vi "Tclk FGV.vi"(8 "Action":T1(ring), 9 "Options":T5={"GetInfo"=TRUE, "Set Det A para"=TRUE, "Set WD"=FALSE, "Set Mag"=TRUE, "Set stig"=FALSE, "Set aln"=FALSE, "Display"=TRUE, "Save"=TRUE, "8-bit"=TRUE, "Detector A"=TRUE, "Detector B"=TRUE, "Detector C"=FALSE, "Detector D"=FALSE, "Inverse A"=FALSE, "Inverse B"=FALSE, "Inverse C"=FALSE, "Inverse D"=FALSE, "Inverse PNG"=FALSE, "Freeze"=TRUE, "PNG only"=FALSE, "Upload"=FALSE, "Delete after upload"=FALSE}, 10 "Scan Para":T3={"X resolution"=0, "Y resolution"=0, "X center (um)"=0.0, "Y center (um)"=0.0, "X size (V)"=0.0, "X size auto"=TRUE, "X stig"=0.0, "Y stig"=0.0, "X aln"=0.0, "Y aln"=0.0, "Scan rate (Hz)"=0, "Oversampling"=0, "Oversampling auto"=TRUE, "Frame line rampdown ratio"=0.0, "Pixel size (nm)"=0.0, "WD"=0.0} {"WD" format="%#_7g"; "Frame line rampdown ratio" min=-1 max=1 step=0.05 format="%.2g"; "Scan rate (Hz)" max=4000000 format="%.2e"}, 11 "HW Config":T4={"SEM X coil"="", "SEM Y coil"="", "Detectors"="", "Det min (V)"=-10.0, "Det max (V)"=10.0, "Eanable COM"=TRUE, "COM port"="", "Detector FIB-NI auto switch"="", "Machine Type"=0, "Machine ID"=""} {"Machine Type" items=["Feiss", "NVision"]}) -> (0 "Tclk handle valid":bool, 3 "Initialized handles":T2={"sessions out"=[], "SEM-X handle out"="", "SEM-Y handle out"="", "SEM-Y waveform handle out"=0, "Detectors handle out"="", "channels"="", "error out"={"status"=FALSE, "code"=0, "source"=""}, "Others"={"AO SampClk.MaxRate"=100000000.0, "AI SampClk.MaxRate"=100000000.0, "AO rate"=10000000.0, "Scan speed"=1, "Detector number"=2, "X min (V)"=-10.0, "X max (V)"=10.0, "X min index"=0, "X max index"=4095, "Y min (V)"=-10.0, "Y max (V)"=10.0, "AO multiline"=128, "Decimating factor"=8, "Total time"=0.9240575999999999, "Scan time (m)"=0.0, "Scan time (s)"=0.9240575999999999, "X resolution"=4096, "Y resolution"=2048, "X resolution with rampdown"=4512, "Oversampling"=10, "Y scan pts per line"=0, "Y scan pts per AO multiline"=0, "Small scan"=FALSE, "Y single line pattern"=[], "Detectors min record length"=0, "Waveform blocks"=16, "Repeat count"=1, "Waveform size"=1155072, "AI multiline"=256}} {"Others"."Scan time (s)" format="%.3f"; "Others"."Scan speed" scale=1.0..15.0; "Others"."AO rate" format="%#_3e"})   [LabVIEW 2018]
uses:
  <instrlib>/niFgen/niFgen.llb/niFgen Output Mode.ctl
  <instrlib>/niScope/Configure/Trigger/niScope Configure Trigger Software.vi
  <instrlib>/niFgen/niFgen.llb/niFgen Write Waveform.vi
  <instrlib>/niFgen/niFgen.llb/niFgen Create Waveform (DBL).vi
  <vilib>/regexp/Match Regular Expression.xnode
panel:
  out "Y min (V)":dbl=-10.0
  out "Y max (V)":dbl=10.0
  out "Detector number":u8=2
  out "X min index":i32
  out "X min (V)":dbl=-10.0
  out "X max index":i32=4095
  out "X max (V)":dbl=10.0
  out "Detector A":bool=TRUE
  out "Detector B":bool=TRUE
  out "Decimating factor":u16=8
  in  "Image fit to":u8(ring) items=["Width", "Height"]
  out "AO multiline":u32=128
  out "Total time":dbl=0.9240575999999999
  out "Y scan pattern":dbl[](array[numeric])
  out "Scan speed":u8(slide)=1 scale=1.0..15.0
  out "Scan time (s)":dbl=0.9240575999999999 format="%.3f"
  out "Scan time (m)":dbl
  out "AI multiline":u16=256
  out "Waveform size":u32=1155072
  out "Repeat count":u32=1
  out "Waveform blocks":u32=16
  out "Small scan":bool
  out "AI SampClk.MaxRate":dbl=100000000.0
  out "AO SampClk.MaxRate":dbl=100000000.0
  out "COM port":refnum<visa-resource-name>="COM1"
  out "X resolution":u32=4096
  out "Y resolution":u32=2048
  out "Scan rate (Hz)":u32=10000000
  out "Oversampling":u32=10
  out "Frame line rampdown ratio":sgl=0.1
  out "Pixel size (nm)":sgl=5.0
  out "WD":sgl=4.0
  out "Det min (V)":dbl=-10.0
  out "Det max (V)":dbl=10.0
  out "X stig":sgl
  out "Y stig":sgl
  out "Detector FIB-NI auto switch":tag="FIB/port0/line0"
  out "SEM X coil":refnum<k15>="SEM-X"
  out "SEM Y coil":refnum<k15>="SEM-Y"
  out "Detectors":refnum<k15>="Detectors"
  out "Y scan rate factor":u8=8
  out "Gain":dbl=10.0
  out "X resolution with rampdown":i32=4512
  out "X single line pattern":dbl[](graph)
  out "Y single line pattern":dbl[](graph)=[-0.5, -0.49951148021494873, -0.4990229604298974, -0.4985344406448461, -0.4980459208597948, -0.49755740107474355, -0.49706888128969223, -0.4965803615046409, -0.49609184171958964, -0.4956033219345384, -0.49511480214948705, -0.49462628236443573, -0.49413776257938447, -0.4936492427943332, -0.4931607230092819, -0.49267220322423055, -0.4921836834391793, -0.491695163654128, -0.4912066438690767, -0.4907181240840254, -0.4902296042989741, -0.48974108451392284, -0.4892525647288715, -0.4887640449438202, -0.48827552515876893, -0.48778700537371766, -0.48729848558866634, -0.486809965803615, -0.48632144601856375, -0.4858329262335125, -0.48534440644846116, -0.48485588666340984, -0.4843673668783586, -0.4838788470933073, -0.483390327308256, -0.48290180752320466, -0.4824132877381534, -0.48192476795310213, -0.4814362481680508, -0.4809477283829995, -0.4804592085979482, -0.47997068881289695, -0.47948216902784563, -0.4789936492427943, -0.47850512945774304, -0.4780166096726918, -0.47752808988764045, -0.4770395701025891, -0.47655105031753786, -0.4760625305324866, -0.47557401074743527, -0.47508549096238395, -0.4745969711773327, -0.4741084513922814, -0.4736199316072301, -0.47313141182217877, -0.4726428920371275, -0.47215437225207624, -0.4716658524670249, -0.4711773326819736, -0.4706888128969223, -0.47020029311187106, -0.46971177332681974, -0.4692232535417684, -0.46873473375671715, -0.4682462139716659, -0.46775769418661456, -0.46726917440156324, -0.46678065461651197, -0.4662921348314607, -0.4658036150464094, -0.46531509526135806, -0.4648265754763068, -0.4643380556912555, -0.4638495359062042, -0.4633610161211529, -0.4628724963361016, -0.46238397655105035, -0.461895456765999, -0.4614069369809477, -0.46091841719589643, -0.46042989741084517, -0.45994137762579385, -0.4594528578407425, -0.45896433805569126, -0.45847581827064, -0.45798729848558867, -0.45749877870053735, -0.4570102589154861, -0.4565217391304348, -0.4560332193453835, -0.45554469956033217, -0.4550561797752809, -0.45456765999022963, -0.4540791402051783, -0.453590620420127, -0.4531021006350757, -0.45261358085002446, -0.45212506106497313, -0.4516365412799218, -0.45114802149487054, -0.4506595017098193, -0.45017098192476795, -0.44968246213971663, -0.44919394235466537, -0.4487054225696141, -0.4482169027845628, -0.44772838299951145, -0.4472398632144602, -0.4467513434294089, -0.4462628236443576, -0.4457743038593063, -0.445285784074255, -0.44479726428920374, -0.4443087445041524, -0.4438202247191011, -0.44333170493404983, -0.44284318514899856, -0.44235466536394724, -0.4418661455788959, -0.44137762579384465, -0.4408891060087934, -0.44040058622374206, -0.43991206643869074, -0.4394235466536395, -0.4389350268685882, -0.4384465070835369, -0.43795798729848556, -0.4374694675134343, -0.43698094772838303, -0.4364924279433317, -0.4360039081582804, -0.4355153883732291, -0.43502686858817785, -0.43453834880312653, -0.4340498290180752, -0.43356130923302394, -0.4330727894479727, -0.43258426966292135, -0.43209574987787003, -0.43160723009281876, -0.4311187103077675, -0.43063019052271617, -0.43014167073766485, -0.4296531509526136, -0.4291646311675623, -0.428676111382511, -0.42818759159745967, -0.4276990718124084, -0.42721055202735714, -0.4267220322423058, -0.4262335124572545, -0.4257449926722032, -0.42525647288715196, -0.42476795310210064, -0.4242794333170493, -0.42379091353199805, -0.4233023937469468, -0.42281387396189546, -0.42232535417684414, -0.42183683439179287, -0.4213483146067416, -0.4208597948216903, -0.42037127503663896, -0.4198827552515877, -0.4193942354665364, -0.4189057156814851, -0.4184171958964338, -0.4179286761113825, -0.41744015632633125, -0.4169516365412799, -0.4164631167562286, -0.41597459697117734, -0.41548607718612607, -0.41499755740107475, -0.4145090376160234, -0.41402051783097216, -0.4135319980459209, -0.41304347826086957, -0.41255495847581825, -0.412066438690767, -0.4115779189057157, -0.4110893991206644, -0.41060087933561307, -0.4101123595505618, -0.40962383976551053, -0.4091353199804592, -0.4086468001954079, -0.4081582804103566, -0.40766976062530536, -0.40718124084025403, -0.4066927210552027, -0.40620420127015144, -0.4057156814851002, -0.40522716170004885, -0.40473864191499753, -0.40425012212994627, -0.403761602344895, -0.4032730825598437, -0.40278456277479235, -0.4022960429897411, -0.4018075232046898, -0.4013190034196385, -0.4008304836345872, -0.4003419638495359, -0.39985344406448464, -0.3993649242794333, -0.398876404494382, -0.39838788470933073, -0.39789936492427946, -0.39741084513922814, -0.3969223253541768, -0.39643380556912555, -0.3959452857840743, -0.39545676599902296, -0.39496824621397164, -0.3944797264289204, -0.3939912066438691, -0.3935026868588178, -0.39301416707376646, -0.3925256472887152, -0.39203712750366393, -0.3915486077186126, -0.3910600879335613, -0.39057156814851, -0.39008304836345875, -0.38959452857840743, -0.3891060087933561, -0.38861748900830484, -0.3881289692232536, -0.38764044943820225, -0.38715192965315093, -0.38666340986809966, -0.3861748900830484, -0.38568637029799707, -0.38519785051294575, -0.3847093307278945, -0.3842208109428432, -0.3837322911577919, -0.38324377137274057, -0.3827552515876893, -0.38226673180263804, -0.3817782120175867, -0.3812896922325354, -0.3808011724474841, -0.38031265266243286, -0.37982413287738154, -0.3793356130923302, -0.37884709330727895, -0.3783585735222277, -0.37787005373717636, -0.37738153395212504, -0.37689301416707377, -0.3764044943820225, -0.3759159745969712, -0.37542745481191986, -0.3749389350268686, -0.3744504152418173, -0.373961895456766, -0.3734733756717147, -0.3729848558866634, -0.37249633610161215, -0.3720078163165608, -0.3715192965315095, -0.37103077674645824, -0.37054225696140697, -0.37005373717635565, -0.3695652173913043, -0.36907669760625306, -0.3685881778212018, -0.36809965803615047, -0.36761113825109915, -0.3671226184660479, -0.3666340986809966, -0.3661455788959453, -0.36565705911089397, -0.3651685393258427, -0.36468001954079143, -0.3641914997557401, -0.3637029799706888, -0.3632144601856375, -0.36272594040058626, -0.36223742061553493, -0.3617489008304836, -0.36126038104543234, -0.3607718612603811, -0.36028334147532975, -0.35979482169027843, -0.35930630190522717, -0.3588177821201759, -0.3583292623351246, -0.35784074255007325, -0.357352222765022, -0.3568637029799707, -0.3563751831949194, -0.3558866634098681, -0.3553981436248168, -0.35490962383976554, -0.3544211040547142, -0.3539325842696629, -0.35344406448461163, -0.35295554469956036, -0.35246702491450904, -0.3519785051294577, -0.35148998534440645, -0.3510014655593552, -0.35051294577430386, -0.35002442598925254, -0.3495359062042013, -0.34904738641915, -0.3485588666340987, -0.34807034684904736, -0.3475818270639961, -0.34709330727894483, -0.3466047874938935, -0.3461162677088422, -0.3456277479237909, -0.34513922813873965, -0.34465070835368833, -0.344162188568637, -0.34367366878358574, -0.3431851489985345, -0.34269662921348315, -0.34220810942843183, -0.34171958964338056, -0.3412310698583293, -0.34074255007327797, -0.34025403028822665, -0.3397655105031754, -0.3392769907181241, -0.3387884709330728, -0.33829995114802147, -0.3378114313629702, -0.33732291157791894, -0.3368343917928676, -0.3363458720078163, -0.335857352222765, -0.33536883243771376, -0.33488031265266244, -0.3343917928676111, -0.33390327308255985, -0.3334147532975086, -0.33292623351245726, -0.33243771372740594, -0.33194919394235467, -0.3314606741573034, -0.3309721543722521, -0.33048363458720076, -0.3299951148021495, -0.3295065950170982, -0.3290180752320469, -0.3285295554469956, -0.3280410356619443, -0.32755251587689305, -0.3270639960918417, -0.3265754763067904, -0.32608695652173914, -0.32559843673668787, -0.32510991695163655, -0.3246213971665852, -0.32413287738153396, -0.3236443575964827, -0.32315583781143137, -0.32266731802638005, -0.3221787982413288, -0.3216902784562775, -0.3212017586712262, -0.32071323888617487, -0.3202247191011236, -0.31973619931607233, -0.319247679531021, -0.3187591597459697, -0.3182706399609184, -0.31778212017586716, -0.31729360039081583, -0.3168050806057645, -0.31631656082071324, -0.315828041035662, -0.31533952125061065, -0.31485100146555933, -0.31436248168050807, -0.3138739618954568, -0.3133854421104055, -0.31289692232535415, -0.3124084025403029, -0.3119198827552516, -0.3114313629702003, -0.310942843185149, -0.3104543234000977, -0.30996580361504644, -0.3094772838299951, -0.3089887640449438, -0.30850024425989253, -0.30801172447484126, -0.30752320468978994, -0.3070346849047386, -0.30654616511968735, -0.3060576453346361, -0.30556912554958476, -0.30508060576453344, -0.3045920859794822, -0.3041035661944309, -0.3036150464093796, -0.30312652662432826, -0.302638006839277, -0.30214948705422573, -0.3016609672691744, -0.3011724474841231, -0.3006839276990718, -0.30019540791402055, -0.29970688812896923, -0.2992183683439179, -0.29872984855886664, -0.2982413287738154, -0.29775280898876405, -0.29726428920371273, -0.29677576941866146, -0.2962872496336102, -0.2957987298485589, -0.29531021006350755, -0.2948216902784563, -0.294333170493405, -0.2938446507083537, -0.29335613092330237, -0.2928676111382511, -0.29237909135319984, -0.2918905715681485, -0.2914020517830972, -0.2909135319980459, -0.29042501221299466, -0.28993649242794334, -0.289447972642892, -0.28895945285784075, -0.2884709330727895, -0.28798241328773816, -0.28749389350268684, -0.28700537371763557, -0.2865168539325843, -0.286028334147533, -0.28553981436248166, -0.2850512945774304, -0.2845627747923791, -0.2840742550073278, -0.2835857352222765, -0.2830972154372252, -0.28260869565217395, -0.2821201758671226, -0.2816316560820713, -0.28114313629702004, -0.28065461651196877, -0.28016609672691745, -0.2796775769418661, -0.27918905715681486, -0.2787005373717636, -0.27821201758671227, -0.27772349780166095, -0.2772349780166097, -0.2767464582315584, -0.2762579384465071, -0.27576941866145577, -0.2752808988764045, -0.27479237909135323, -0.2743038593063019, -0.2738153395212506, -0.2733268197361993, -0.27283829995114806, -0.27234978016609673, -0.2718612603810454, -0.27137274059599414, -0.2708842208109429, -0.27039570102589155, -0.26990718124084023, -0.26941866145578897, -0.2689301416707377, -0.2684416218856864, -0.26795310210063505, -0.2674645823155838, -0.2669760625305325, -0.2664875427454812, -0.2659990229604299, -0.2655105031753786, -0.26502198339032734, -0.264533463605276, -0.2640449438202247, -0.26355642403517343, -0.26306790425012216, -0.26257938446507084, -0.2620908646800195, -0.26160234489496825, -0.261113825109917, -0.26062530532486566, -0.26013678553981434, -0.2596482657547631, -0.2591597459697118, -0.2586712261846605, -0.25818270639960916, -0.2576941866145579, -0.25720566682950663, -0.2567171470444553, -0.256228627259404, -0.2557401074743527, -0.25525158768930145, -0.25476306790425013, -0.2542745481191988, -0.25378602833414754, -0.2532975085490963, -0.25280898876404495, -0.25232046897899363, -0.25183194919394236, -0.2513434294088911, -0.2508549096238398, -0.25036638983878845, -0.24987787005373718, -0.24938935026868592, -0.2489008304836346, -0.24841231069858327, -0.247923790913532, -0.24743527112848074, -0.24694675134342942, -0.2464582315583781, -0.24596971177332683, -0.24548119198827556, -0.24499267220322424, -0.24450415241817292, -0.24401563263312165, -0.24352711284807038, -0.24303859306301906, -0.24255007327796774, -0.24206155349291647, -0.2415730337078652, -0.24108451392281388, -0.24059599413776256, -0.2401074743527113, -0.23961895456766003, -0.2391304347826087, -0.23864191499755738, -0.2381533952125061, -0.23766487542745485, -0.23717635564240352, -0.2366878358573522, -0.23619931607230094, -0.23571079628724967, -0.23522227650219835, -0.23473375671714702, -0.23424523693209576, -0.2337567171470445, -0.23326819736199317, -0.23277967757694185, -0.23229115779189058, -0.2318026380068393, -0.231314118221788, -0.23082559843673667, -0.2303370786516854, -0.22984855886663413, -0.2293600390815828, -0.2288715192965315, -0.22838299951148022, -0.22789447972642896, -0.22740595994137763, -0.2269174401563263, -0.22642892037127504, -0.22594040058622378, -0.22545188080117246, -0.22496336101612113, -0.22447484123106987, -0.2239863214460186, -0.22349780166096728, -0.22300928187591595, -0.2225207620908647, -0.22203224230581342, -0.2215437225207621, -0.22105520273571078, -0.2205666829506595, -0.22007816316560824, -0.21958964338055692, -0.2191011235955056, -0.21861260381045433, -0.21812408402540306, -0.21763556424035174, -0.21714704445530042, -0.21665852467024915, -0.2161700048851979, -0.21568148510014656, -0.21519296531509524, -0.21470444553004397, -0.2142159257449927, -0.21372740595994139, -0.21323888617489006, -0.2127503663898388, -0.21226184660478753, -0.2117733268197362, -0.21128480703468488, -0.21079628724963362, -0.21030776746458235, -0.20981924767953103, -0.2093307278944797, -0.20884220810942844, -0.20835368832437717, -0.20786516853932585, -0.20737664875427453, -0.20688812896922326, -0.206399609184172, -0.20591108939912067, -0.20542256961406935, -0.20493404982901808, -0.20444553004396682, -0.2039570102589155, -0.20346849047386417, -0.2029799706888129, -0.20249145090376164, -0.20200293111871032, -0.201514411333659, -0.20102589154860773, -0.20053737176355646, -0.20004885197850514, -0.19956033219345382, -0.19907181240840255, -0.19858329262335128, -0.19809477283829996, -0.19760625305324864, -0.19711773326819737, -0.1966292134831461, -0.19614069369809478, -0.19565217391304346, -0.1951636541279922, -0.19467513434294093, -0.1941866145578896, -0.19369809477283828, -0.19320957498778701, -0.19272105520273575, -0.19223253541768442, -0.1917440156326331, -0.19125549584758184, -0.19076697606253057, -0.19027845627747925, -0.18978993649242792, -0.18930141670737666, -0.1888128969223254, -0.18832437713727407, -0.18783585735222275, -0.18734733756717148, -0.1868588177821202, -0.1863702979970689, -0.18588177821201757, -0.1853932584269663, -0.18490473864191503, -0.1844162188568637, -0.1839276990718124, -0.18343917928676112, -0.18295065950170986, -0.18246213971665853, -0.1819736199316072, -0.18148510014655594, -0.18099658036150468, -0.18050806057645336, -0.18001954079140203, -0.17953102100635077, -0.1790425012212995, -0.17855398143624818, -0.17806546165119685, -0.1775769418661456, -0.17708842208109432, -0.176599902296043, -0.17611138251099168, -0.1756228627259404, -0.17513434294088914, -0.17464582315583782, -0.1741573033707865, -0.17366878358573523, -0.17318026380068396, -0.17269174401563264, -0.17220322423058132, -0.17171470444553005, -0.1712261846604788, -0.17073766487542746, -0.17024914509037614, -0.16976062530532487, -0.1692721055202736, -0.16878358573522229, -0.16829506595017096, -0.1678065461651197, -0.16731802638006843, -0.1668295065950171, -0.16634098680996579, -0.16585246702491452, -0.16536394723986325, -0.16487542745481193, -0.1643869076697606, -0.16389838788470934, -0.16340986809965807, -0.16292134831460675, -0.16243282852955543, -0.16194430874450416, -0.1614557889594529, -0.16096726917440157, -0.16047874938935025, -0.15999022960429898, -0.15950170981924772, -0.1590131900341964, -0.15852467024914507, -0.1580361504640938, -0.15754763067904254, -0.15705911089399122, -0.1565705911089399, -0.15608207132388863, -0.15559355153883736, -0.15510503175378604, -0.15461651196873472, -0.15412799218368345, -0.15363947239863218, -0.15315095261358086, -0.15266243282852954, -0.15217391304347827, -0.151685393258427, -0.15119687347337568, -0.15070835368832436, -0.1502198339032731, -0.14973131411822183, -0.1492427943331705, -0.14875427454811918, -0.14826575476306791, -0.14777723497801665, -0.14728871519296532, -0.146800195407914, -0.14631167562286274, -0.14582315583781147, -0.14533463605276015, -0.14484611626770882, -0.14435759648265756, -0.1438690766976063, -0.14338055691255497, -0.14289203712750365, -0.14240351734245238, -0.1419149975574011, -0.1414264777723498, -0.14093795798729847, -0.1404494382022472, -0.13996091841719593, -0.1394723986321446, -0.1389838788470933, -0.13849535906204202, -0.13800683927699076, -0.13751831949193943, -0.1370297997068881, -0.13654127992183684, -0.13605276013678558, -0.13556424035173426, -0.13507572056668293, -0.13458720078163167, -0.1340986809965804, -0.13361016121152908, -0.13312164142647775, -0.1326331216414265, -0.13214460185637522, -0.1316560820713239, -0.13116756228627258, -0.1306790425012213, -0.13019052271617004, -0.12970200293111872, -0.1292134831460674, -0.12872496336101613, -0.12823644357596486, -0.12774792379091354, -0.12725940400586222, -0.12677088422081095, -0.1262823644357597, -0.12579384465070836, -0.12530532486565704, -0.12481680508060577, -0.12432828529555451, -0.12383976551050319, -0.12335124572545186, -0.1228627259404006, -0.12237420615534933, -0.12188568637029801, -0.12139716658524669, -0.12090864680019542, -0.12042012701514415, -0.11993160723009283, -0.11944308744504151, -0.11895456765999024, -0.11846604787493897, -0.11797752808988765, -0.11748900830483633, -0.11700048851978506, -0.1165119687347338, -0.11602344894968247, -0.11553492916463115, -0.11504640937957988, -0.11455788959452862, -0.1140693698094773, -0.11358085002442597, -0.1130923302393747, -0.11260381045432344, -0.11211529066927212, -0.1116267708842208, -0.11113825109916953, -0.11064973131411826, -0.11016121152906694, -0.10967269174401562, -0.10918417195896435, -0.10869565217391308, -0.10820713238886176, -0.10771861260381044, -0.10723009281875917, -0.1067415730337079, -0.10625305324865658, -0.10576453346360526, -0.10527601367855399, -0.10478749389350273, -0.1042989741084514, -0.10381045432340008, -0.10332193453834881, -0.10283341475329755, -0.10234489496824623, -0.1018563751831949, -0.10136785539814364, -0.10087933561309237, -0.10039081582804105, -0.09990229604298972, -0.09941377625793846, -0.09892525647288719, -0.09843673668783587, -0.09794821690278455, -0.09745969711773328, -0.09697117733268201, -0.09648265754763069, -0.09599413776257937, -0.0955056179775281, -0.09501709819247683, -0.09452857840742551, -0.09404005862237419, -0.09355153883732292, -0.09306301905227166, -0.09257449926722033, -0.09208597948216901, -0.09159745969711774, -0.09110893991206648, -0.09062042012701516, -0.09013190034196383, -0.08964338055691257, -0.0891548607718613, -0.08866634098680998, -0.08817782120175865, -0.08768930141670739, -0.08720078163165612, -0.0867122618466048, -0.08622374206155348, -0.08573522227650221, -0.08524670249145094, -0.08475818270639962, -0.0842696629213483, -0.08378114313629703, -0.08329262335124576, -0.08280410356619444, -0.08231558378114312, -0.08182706399609185, -0.08133854421104059, -0.08085002442598926, -0.08036150464093794, -0.07987298485588668, -0.07938446507083541, -0.07889594528578409, -0.07840742550073276, -0.0779189057156815, -0.07743038593063023, -0.07694186614557891, -0.07645334636052759, -0.07596482657547632, -0.07547630679042505, -0.07498778700537373, -0.07449926722032241, -0.07401074743527114, -0.07352222765021987, -0.07303370786516855, -0.07254518808011723, -0.07205666829506596, -0.0715681485100147, -0.07107962872496337, -0.07059110893991205, -0.07010258915486078, -0.06961406936980952, -0.0691255495847582, -0.06863702979970687, -0.0681485100146556, -0.06765999022960434, -0.06717147044455302, -0.0666829506595017, -0.06619443087445043, -0.06570591108939916, -0.06521739130434784, -0.06472887151929652, -0.06424035173424525, -0.06375183194919398, -0.06326331216414266, -0.06277479237909134, -0.06228627259404007, -0.061797752808988804, -0.06130923302393748, -0.06082071323888616, -0.06033219345383489, -0.059843673668783626, -0.0593551538837323, -0.05886663409868098, -0.058378114313629714, -0.05788959452857845, -0.057401074743527125, -0.0569125549584758, -0.056424035173424536, -0.05593551538837327, -0.05544699560332195, -0.054958475818270625, -0.05446995603321936, -0.05398143624816809, -0.05349291646311677, -0.053004396678065446, -0.05251587689301418, -0.05202735710796291, -0.05153883732291159, -0.05105031753786027, -0.050561797752809, -0.050073277967757734, -0.04958475818270641, -0.04909623839765509, -0.04860771861260382, -0.048119198827552556, -0.047630679042501234, -0.04714215925744991, -0.046653639472398645, -0.04616511968734738, -0.045676599902296056, -0.04518808011724473, -0.044699560332193466, -0.0442110405471422, -0.04372252076209088, -0.043234000977039555, -0.04274548119198829, -0.04225696140693702, -0.0417684416218857, -0.04127992183683438, -0.04079140205178311, -0.04030288226673184, -0.03981436248168052, -0.0393258426966292, -0.03883732291157793, -0.038348803126526665, -0.03786028334147534, -0.03737176355642402, -0.03688324377137275, -0.03639472398632149, -0.035906204201270164, -0.03541768441621884, -0.034929164631167575, -0.03444064484611631, -0.033952125061064986, -0.033463605276013664, -0.0329750854909624, -0.03248656570591113, -0.03199804592085981, -0.031509526135808485, -0.03102100635075722, -0.030532486565705952, -0.03004396678065463, -0.029555446995603307, -0.02906692721055204, -0.028578407425500774, -0.02808988764044945, -0.02760136785539813, -0.027112848070346862, -0.026624328285295595, -0.026135808500244273, -0.02564728871519295, -0.025158768930141684, -0.024670249145090417, -0.024181729360039095, -0.023693209574987772, -0.023204689789936506, -0.02271617000488524, -0.022227650219833917, -0.021739130434782594, -0.021250610649731327, -0.02076209086468006, -0.02027357107962874, -0.019785051294577416, -0.01929653150952615, -0.018808011724474882, -0.01831949193942356, -0.017830972154372238, -0.01734245236932097, -0.016853932584269704, -0.016365412799218382, -0.01587689301416706, -0.015388373229115793, -0.014899853444064526, -0.014411333659013204, -0.013922813873961881, -0.013434294088910614, -0.012945774303859348, -0.012457254518808025, -0.011968734733756703, -0.011480214948705436, -0.01099169516365417, -0.010503175378602847, -0.010014655593551525, -0.009526135808500258, -0.009037616023448991, -0.008549096238397669, -0.008060576453346346, -0.00757205666829508, -0.007083536883243813, -0.0065950170981924905, -0.006106497313141168, -0.005617977528089901, -0.0051294577430386346, -0.004640937957987312, -0.00415241817293599, -0.003663898387884723, -0.0031753786028334563, -0.002686858817782134, -0.0021983390327308117, -0.0017098192476795449, -0.001221299462628278, -0.0007327796775769557, -0.0002442598925256334, 0.0002442598925256334, 0.0007327796775769002, 0.001221299462628167, 0.0017098192476795449, 0.0021983390327308117, 0.0026868588177820785, 0.0031753786028334563, 0.003663898387884723, 0.00415241817293599, 0.004640937957987257, 0.0051294577430385235, 0.005617977528089901, 0.006106497313141168, 0.006595017098192435, 0.007083536883243813, 0.00757205666829508, 0.008060576453346346, 0.008549096238397613, 0.00903761602344888, 0.009526135808500258, 0.010014655593551525, 0.010503175378602791, 0.01099169516365417, 0.011480214948705436, 0.011968734733756703, 0.01245725451880797, 0.012945774303859237, 0.013434294088910614, 0.013922813873961881, 0.014411333659013148, 0.014899853444064526, 0.015388373229115793, 0.01587689301416706, 0.016365412799218326, 0.016853932584269593, 0.01734245236932097, 0.017830972154372238, 0.018319491939423505, 0.018808011724474882, 0.01929653150952615, 0.019785051294577416, 0.020273571079628683, 0.02076209086467995, 0.021250610649731327, 0.021739130434782594, 0.02222765021983386, 0.02271617000488524, 0.023204689789936506, 0.023693209574987772, 0.02418172936003904, 0.024670249145090306, 0.025158768930141684, 0.02564728871519295, 0.026135808500244218, 0.026624328285295595, 0.027112848070346862, 0.02760136785539813, 0.028089887640449396, 0.028578407425500663, 0.02906692721055204, 0.029555446995603307, 0.030043966780654574, 0.030532486565705952, 0.03102100635075722, 0.031509526135808485, 0.03199804592085975, 0.03248656570591102, 0.0329750854909624, 0.033463605276013664, 0.03395212506106493, 0.03444064484611631, 0.034929164631167575, 0.03541768441621884, 0.03590620420127011, 0.036394723986321376, 0.03688324377137275, 0.03737176355642402, 0.03786028334147529, 0.038348803126526665, 0.03883732291157793, 0.0393258426966292, 0.039814362481680465, 0.04030288226673173, 0.04079140205178311, 0.04127992183683438, 0.041768441621885644, 0.04225696140693702, 0.04274548119198829, 0.043234000977039555, 0.04372252076209082, 0.04421104054714209, 0.044699560332193466, 0.04518808011724473, 0.045676599902296, 0.04616511968734738, 0.046653639472398645, 0.04714215925744991, 0.04763067904250118, 0.048119198827552445, 0.04860771861260382, 0.04909623839765509, 0.04958475818270636, 0.050073277967757734, 0.050561797752809, 0.05105031753786027, 0.051538837322911535, 0.0520273571079628, 0.05251587689301418, 0.053004396678065446, 0.05349291646311671, 0.05398143624816809, 0.05446995603321936, 0.054958475818270625, 0.05544699560332189, 0.05593551538837316, 0.056424035173424536, 0.0569125549584758, 0.05740107474352707, 0.05788959452857845, 0.058378114313629714, 0.05886663409868098, 0.05935515388373225, 0.059843673668783515, 0.06033219345383489, 0.06082071323888616, 0.061309233023937426, 0.061797752808988804, 0.06228627259404007, 0.06277479237909134, 0.0632633121641426, 0.06375183194919387, 0.06424035173424525, 0.06472887151929652, 0.06521739130434778, 0.06570591108939916, 0.06619443087445043, 0.0666829506595017, 0.06717147044455296, 0.06765999022960423, 0.0681485100146556, 0.06863702979970687, 0.06912554958475814, 0.06961406936980952, 0.07010258915486078, 0.07059110893991205, 0.07107962872496332, 0.07156814851001458, 0.07205666829506596, 0.07254518808011723, 0.0730337078651685, 0.07352222765021987, 0.07401074743527114, 0.07449926722032241, 0.07498778700537367, 0.07547630679042494, 0.07596482657547632, 0.07645334636052759, 0.07694186614557885, 0.07743038593063023, 0.0779189057156815, 0.07840742550073276, 0.07889594528578403, 0.0793844650708353, 0.07987298485588668, 0.08036150464093794, 0.08085002442598921, 0.08133854421104059, 0.08182706399609185, 0.08231558378114312, 0.08280410356619439, 0.08329262335124565, 0.08378114313629703, 0.0842696629213483, 0.08475818270639957, 0.08524670249145094, 0.08573522227650221, 0.08622374206155348, 0.08671226184660474, 0.08720078163165601, 0.08768930141670739, 0.08817782120175865, 0.08866634098680992, 0.0891548607718613, 0.08964338055691257, 0.09013190034196383, 0.0906204201270151, 0.09110893991206637, 0.09159745969711774, 0.09208597948216901, 0.09257449926722028, 0.09306301905227166, 0.09355153883732292, 0.09404005862237419, 0.09452857840742546, 0.09501709819247672, 0.0955056179775281, 0.09599413776257937, 0.09648265754763063, 0.09697117733268201, 0.09745969711773328, 0.09794821690278455, 0.09843673668783581, 0.09892525647288708, 0.09941377625793846, 0.09990229604298972, 0.10039081582804099, 0.10087933561309237, 0.10136785539814364, 0.1018563751831949, 0.10234489496824617, 0.10283341475329744, 0.10332193453834881, 0.10381045432340008, 0.10429897410845135, 0.10478749389350273, 0.10527601367855399, 0.10576453346360526, 0.10625305324865653, 0.10674157303370779, 0.10723009281875917, 0.10771861260381044, 0.1082071323888617, 0.10869565217391308, 0.10918417195896435, 0.10967269174401562, 0.11016121152906688, 0.11064973131411815, 0.11113825109916953, 0.1116267708842208, 0.11211529066927206, 0.11260381045432344, 0.1130923302393747, 0.11358085002442597, 0.11406936980947724, 0.1145578895945285, 0.11504640937957988, 0.11553492916463115, 0.11602344894968242, 0.1165119687347338, 0.11700048851978506, 0.11748900830483633, 0.1179775280898876, 0.11846604787493886, 0.11895456765999024, 0.11944308744504151, 0.11993160723009277, 0.12042012701514415, 0.12090864680019542, 0.12139716658524669, 0.12188568637029795, 0.12237420615534922, 0.1228627259404006, 0.12335124572545186, 0.12383976551050313, 0.12432828529555451, 0.12481680508060577, 0.12530532486565704, 0.1257938446507083, 0.12628236443575958, 0.12677088422081095, 0.12725940400586222, 0.1277479237909135, 0.12823644357596486, 0.12872496336101613, 0.1292134831460674, 0.12970200293111867, 0.13019052271616993, 0.1306790425012213, 0.13116756228627258, 0.13165608207132384, 0.13214460185637522, 0.1326331216414265, 0.13312164142647775, 0.13361016121152902, 0.1340986809965803, 0.13458720078163167, 0.13507572056668293, 0.1355642403517342, 0.13605276013678558, 0.13654127992183684, 0.1370297997068881, 0.13751831949193938, 0.13800683927699064, 0.13849535906204202, 0.1389838788470933, 0.13947239863214456, 0.13996091841719593, 0.1404494382022472, 0.14093795798729847, 0.14142647777234973, 0.141914997557401, 0.14240351734245238, 0.14289203712750365, 0.1433805569125549, 0.1438690766976063, 0.14435759648265756, 0.14484611626770882, 0.1453346360527601, 0.14582315583781136, 0.14631167562286274, 0.146800195407914, 0.14728871519296527, 0.14777723497801665, 0.14826575476306791, 0.14875427454811918, 0.14924279433317045, 0.14973131411822171, 0.1502198339032731, 0.15070835368832436, 0.15119687347337563, 0.151685393258427, 0.15217391304347827, 0.15266243282852954, 0.1531509526135808, 0.15363947239863207, 0.15412799218368345, 0.15461651196873472, 0.15510503175378598, 0.15559355153883736, 0.15608207132388863, 0.1565705911089399, 0.15705911089399116, 0.15754763067904243, 0.1580361504640938, 0.15852467024914507, 0.15901319003419634, 0.15950170981924772, 0.15999022960429898, 0.16047874938935025, 0.16096726917440152, 0.16145578895945278, 0.16194430874450416, 0.16243282852955543, 0.1629213483146067, 0.16340986809965807, 0.16389838788470934, 0.1643869076697606, 0.16487542745481187, 0.16536394723986314, 0.16585246702491452, 0.16634098680996579, 0.16682950659501705, 0.16731802638006843, 0.1678065461651197, 0.16829506595017096, 0.16878358573522223, 0.1692721055202735, 0.16976062530532487, 0.17024914509037614, 0.1707376648754274, 0.1712261846604788, 0.17171470444553005, 0.17220322423058132, 0.1726917440156326, 0.17318026380068385, 0.17366878358573523, 0.1741573033707865, 0.17464582315583776, 0.17513434294088914, 0.1756228627259404, 0.17611138251099168, 0.17659990229604294, 0.1770884220810942, 0.1775769418661456, 0.17806546165119685, 0.17855398143624812, 0.1790425012212995, 0.17953102100635077, 0.18001954079140203, 0.1805080605764533, 0.18099658036150457, 0.18148510014655594, 0.1819736199316072, 0.18246213971665848, 0.18295065950170986, 0.18343917928676112, 0.1839276990718124, 0.18441621885686366, 0.18490473864191492, 0.1853932584269663, 0.18588177821201757, 0.18637029799706883, 0.1868588177821202, 0.18734733756717148, 0.18783585735222275, 0.188324377137274, 0.18881289692232528, 0.18930141670737666, 0.18978993649242792, 0.1902784562774792, 0.19076697606253057, 0.19125549584758184, 0.1917440156326331, 0.19223253541768437, 0.19272105520273564, 0.19320957498778701, 0.19369809477283828, 0.19418661455788955, 0.19467513434294093, 0.1951636541279922, 0.19565217391304346, 0.19614069369809473, 0.196629213483146, 0.19711773326819737, 0.19760625305324864, 0.1980947728382999, 0.19858329262335128, 0.19907181240840255, 0.19956033219345382, 0.20004885197850508, 0.20053737176355635, 0.20102589154860773, 0.201514411333659, 0.20200293111871026, 0.20249145090376164, 0.2029799706888129, 0.20346849047386417, 0.20395701025891544, 0.2044455300439667, 0.20493404982901808, 0.20542256961406935, 0.20591108939912062, 0.206399609184172, 0.20688812896922326, 0.20737664875427453, 0.2078651685393258, 0.20835368832437706, 0.20884220810942844, 0.2093307278944797, 0.20981924767953097, 0.21030776746458235, 0.21079628724963362, 0.21128480703468488, 0.21177332681973615, 0.21226184660478742, 0.2127503663898388, 0.21323888617489006, 0.21372740595994133, 0.2142159257449927, 0.21470444553004397, 0.21519296531509524, 0.2156814851001465, 0.21617000488519778, 0.21665852467024915, 0.21714704445530042, 0.2176355642403517, 0.21812408402540306, 0.21861260381045433, 0.2191011235955056, 0.21958964338055686, 0.22007816316560813, 0.2205666829506595, 0.22105520273571078, 0.22154372252076204, 0.22203224230581342, 0.2225207620908647, 0.22300928187591595, 0.22349780166096722, 0.2239863214460185, 0.22447484123106987, 0.22496336101612113, 0.2254518808011724, 0.22594040058622378, 0.22642892037127504, 0.2269174401563263, 0.22740595994137758, 0.22789447972642884, 0.22838299951148022, 0.2288715192965315, 0.22936003908158276, 0.22984855886663413, 0.2303370786516854, 0.23082559843673667, 0.23131411822178793, 0.2318026380068392, 0.23229115779189058, 0.23277967757694185, 0.2332681973619931, 0.2337567171470445, 0.23424523693209576, 0.23473375671714702, 0.2352222765021983, 0.23571079628724956, 0.23619931607230094, 0.2366878358573522, 0.23717635564240347, 0.23766487542745485, 0.2381533952125061, 0.23864191499755738, 0.23913043478260865, 0.23961895456765991, 0.2401074743527113, 0.24059599413776256, 0.24108451392281383, 0.2415730337078652, 0.24206155349291647, 0.24255007327796774, 0.243038593063019, 0.24352711284807027, 0.24401563263312165, 0.24450415241817292, 0.24499267220322418, 0.24548119198827556, 0.24596971177332683, 0.2464582315583781, 0.24694675134342936, 0.24743527112848063, 0.247923790913532, 0.24841231069858327, 0.24890083048363454, 0.24938935026868592, 0.24987787005373718, 0.25036638983878845, 0.2508549096238397, 0.251343429408891, 0.25183194919394236, 0.25232046897899363, 0.2528089887640449, 0.2532975085490963, 0.25378602833414754, 0.2542745481191988, 0.2547630679042501, 0.25525158768930134, 0.2557401074743527, 0.256228627259404, 0.25671714704445525, 0.25720566682950663, 0.2576941866145579, 0.25818270639960916, 0.25867122618466043, 0.2591597459697117, 0.2596482657547631, 0.26013678553981434, 0.2606253053248656, 0.261113825109917, 0.26160234489496825, 0.2620908646800195, 0.2625793844650708, 0.26306790425012205, 0.26355642403517343, 0.2640449438202247, 0.26453346360527596, 0.26502198339032734, 0.2655105031753786, 0.2659990229604299, 0.26648754274548114, 0.2669760625305324, 0.2674645823155838, 0.26795310210063505, 0.2684416218856863, 0.2689301416707377, 0.26941866145578897, 0.26990718124084023, 0.2703957010258915, 0.27088422081094277, 0.27137274059599414, 0.2718612603810454, 0.2723497801660967, 0.27283829995114806, 0.2733268197361993, 0.2738153395212506, 0.27430385930630186, 0.2747923790913531, 0.2752808988764045, 0.27576941866145577, 0.27625793844650703, 0.2767464582315584, 0.2772349780166097, 0.27772349780166095, 0.2782120175867122, 0.2787005373717635, 0.27918905715681486, 0.2796775769418661, 0.2801660967269174, 0.28065461651196877, 0.28114313629702004, 0.2816316560820713, 0.28212017586712257, 0.28260869565217384, 0.2830972154372252, 0.2835857352222765, 0.28407425500732775, 0.2845627747923791, 0.2850512945774304, 0.28553981436248166, 0.2860283341475329, 0.2865168539325842, 0.28700537371763557, 0.28749389350268684, 0.2879824132877381, 0.2884709330727895, 0.28895945285784075, 0.289447972642892, 0.2899364924279433, 0.29042501221299455, 0.2909135319980459, 0.2914020517830972, 0.29189057156814846, 0.29237909135319984, 0.2928676111382511, 0.29335613092330237, 0.29384465070835364, 0.2943331704934049, 0.2948216902784563, 0.29531021006350755, 0.2957987298485588, 0.2962872496336102, 0.29677576941866146, 0.29726428920371273, 0.297752808988764, 0.29824132877381526, 0.29872984855886664, 0.2992183683439179, 0.2997068881289692, 0.30019540791402055, 0.3006839276990718, 0.3011724474841231, 0.30166096726917435, 0.3021494870542256, 0.302638006839277, 0.30312652662432826, 0.30361504640937953, 0.3041035661944309, 0.3045920859794822, 0.30508060576453344, 0.3055691255495847, 0.306057645334636, 0.30654616511968735, 0.3070346849047386, 0.3075232046897899, 0.30801172447484126, 0.30850024425989253, 0.3089887640449438, 0.30947728382999506, 0.30996580361504633, 0.3104543234000977, 0.310942843185149, 0.31143136297020024, 0.3119198827552516, 0.3124084025403029, 0.31289692232535415, 0.3133854421104054, 0.3138739618954567, 0.31436248168050807, 0.31485100146555933, 0.3153395212506106, 0.315828041035662, 0.31631656082071324, 0.3168050806057645, 0.3172936003908158, 0.31778212017586704, 0.3182706399609184, 0.3187591597459697, 0.31924767953102096, 0.31973619931607233, 0.3202247191011236, 0.32071323888617487, 0.32120175867122613, 0.3216902784562774, 0.3221787982413288, 0.32266731802638005, 0.3231558378114313, 0.3236443575964827, 0.32413287738153396, 0.3246213971665852, 0.3251099169516365, 0.32559843673668776, 0.32608695652173914, 0.3265754763067904, 0.32706399609184167, 0.32755251587689305, 0.3280410356619443, 0.3285295554469956, 0.32901807523204685, 0.3295065950170981, 0.3299951148021495, 0.33048363458720076, 0.330972154372252, 0.3314606741573034, 0.33194919394235467, 0.33243771372740594, 0.3329262335124572, 0.33341475329750847, 0.33390327308255985, 0.3343917928676111, 0.3348803126526624, 0.33536883243771376, 0.335857352222765, 0.3363458720078163, 0.33683439179286756, 0.3373229115779188, 0.3378114313629702, 0.33829995114802147, 0.33878847093307274, 0.3392769907181241, 0.3397655105031754, 0.34025403028822665, 0.3407425500732779, 0.3412310698583292, 0.34171958964338056, 0.34220810942843183, 0.3426966292134831, 0.3431851489985345, 0.34367366878358574, 0.344162188568637, 0.3446507083536883, 0.34513922813873954, 0.3456277479237909, 0.3461162677088422, 0.34660478749389345, 0.34709330727894483, 0.3475818270639961, 0.34807034684904736, 0.34855886663409863, 0.3490473864191499, 0.3495359062042013, 0.35002442598925254, 0.3505129457743038, 0.3510014655593552, 0.35148998534440645, 0.3519785051294577, 0.352467024914509, 0.35295554469956025, 0.35344406448461163, 0.3539325842696629, 0.35442110405471416, 0.35490962383976554, 0.3553981436248168, 0.3558866634098681, 0.35637518319491934, 0.3568637029799706, 0.357352222765022, 0.35784074255007325, 0.3583292623351245, 0.3588177821201759, 0.35930630190522717, 0.35979482169027843, 0.3602833414753297, 0.36077186126038097, 0.36126038104543234, 0.3617489008304836, 0.3622374206155349, 0.36272594040058626, 0.3632144601856375, 0.3637029799706888, 0.36419149975574006, 0.3646800195407913, 0.3651685393258427, 0.36565705911089397, 0.36614557889594523, 0.3666340986809966, 0.3671226184660479, 0.36761113825109915, 0.3680996580361504, 0.3685881778212017, 0.36907669760625306, 0.3695652173913043, 0.3700537371763556, 0.37054225696140697, 0.37103077674645824, 0.3715192965315095, 0.37200781631656077, 0.37249633610161204, 0.3729848558866634, 0.3734733756717147, 0.37396189545676595, 0.3744504152418173, 0.3749389350268686, 0.37542745481191986, 0.3759159745969711, 0.3764044943820224, 0.37689301416707377, 0.37738153395212504, 0.3778700537371763, 0.3783585735222277, 0.37884709330727895, 0.3793356130923302, 0.3798241328773815, 0.38031265266243275, 0.3808011724474841, 0.3812896922325354, 0.38177821201758666, 0.38226673180263804, 0.3827552515876893, 0.38324377137274057, 0.38373229115779184, 0.3842208109428431, 0.3847093307278945, 0.38519785051294575, 0.385686370297997, 0.3861748900830484, 0.38666340986809966, 0.38715192965315093, 0.3876404494382022, 0.38812896922325346, 0.38861748900830484, 0.3891060087933561, 0.3895945285784074, 0.39008304836345875, 0.39057156814851, 0.3910600879335613, 0.39154860771861255, 0.3920371275036638, 0.3925256472887152, 0.39301416707376646, 0.39350268685881773, 0.3939912066438691, 0.3944797264289204, 0.39496824621397164, 0.3954567659990229, 0.3959452857840742, 0.39643380556912555, 0.3969223253541768, 0.3974108451392281, 0.39789936492427946, 0.39838788470933073, 0.398876404494382, 0.39936492427943326, 0.39985344406448453, 0.4003419638495359, 0.4008304836345872, 0.40131900341963844, 0.4018075232046898, 0.4022960429897411, 0.40278456277479235, 0.4032730825598436, 0.4037616023448949, 0.40425012212994627, 0.40473864191499753, 0.4052271617000488, 0.4057156814851002, 0.40620420127015144, 0.4066927210552027, 0.407181240840254, 0.40766976062530524, 0.4081582804103566, 0.4086468001954079, 0.40913531998045916, 0.40962383976551053, 0.4101123595505618, 0.41060087933561307, 0.41108939912066433, 0.4115779189057156, 0.412066438690767, 0.41255495847581825, 0.4130434782608695, 0.4135319980459209, 0.41402051783097216, 0.4145090376160234, 0.4149975574010747, 0.41548607718612596, 0.41597459697117734, 0.4164631167562286, 0.41695163654127987, 0.41744015632633125, 0.4179286761113825, 0.4184171958964338, 0.41890571568148505, 0.4193942354665363, 0.4198827552515877, 0.42037127503663896, 0.4208597948216902, 0.4213483146067416, 0.42183683439179287, 0.42232535417684414, 0.4228138739618954, 0.42330239374694667, 0.42379091353199805, 0.4242794333170493, 0.4247679531021006, 0.42525647288715196, 0.4257449926722032, 0.4262335124572545, 0.42672203224230576, 0.427210552027357, 0.4276990718124084, 0.42818759159745967, 0.42867611138251094, 0.4291646311675623, 0.4296531509526136, 0.43014167073766485, 0.4306301905227161, 0.4311187103077674, 0.43160723009281876, 0.43209574987787003, 0.4325842696629213, 0.4330727894479727, 0.43356130923302394, 0.4340498290180752, 0.4345383488031265, 0.43502686858817774, 0.4355153883732291, 0.4360039081582804, 0.43649242794333165, 0.43698094772838303, 0.4374694675134343, 0.43795798729848556, 0.43844650708353683, 0.4389350268685881, 0.4394235466536395, 0.43991206643869074, 0.440400586223742, 0.4408891060087934, 0.44137762579384465, 0.4418661455788959, 0.4423546653639472, 0.44284318514899845, 0.44333170493404983, 0.4438202247191011, 0.44430874450415236, 0.44479726428920374, 0.445285784074255, 0.4457743038593063, 0.44626282364435754, 0.4467513434294088, 0.4472398632144602, 0.44772838299951145, 0.4482169027845627, 0.4487054225696141, 0.44919394235466537, 0.44968246213971663, 0.4501709819247679, 0.45065950170981917, 0.45114802149487054, 0.4516365412799218, 0.4521250610649731, 0.45261358085002446, 0.4531021006350757, 0.453590620420127, 0.45407914020517826, 0.4545676599902295, 0.4550561797752809, 0.45554469956033217, 0.45603321934538343, 0.4565217391304348, 0.4570102589154861, 0.45749877870053735, 0.4579872984855886, 0.4584758182706399, 0.45896433805569126, 0.4594528578407425, 0.4599413776257938, 0.46042989741084517, 0.46091841719589643, 0.4614069369809477, 0.46189545676599897, 0.46238397655105024, 0.4628724963361016, 0.4633610161211529, 0.46384953590620415, 0.4643380556912555, 0.4648265754763068, 0.46531509526135806, 0.4658036150464093, 0.4662921348314606, 0.46678065461651197, 0.46726917440156324, 0.4677576941866145, 0.4682462139716659, 0.46873473375671715, 0.4692232535417684, 0.4697117733268197, 0.47020029311187095, 0.4706888128969223, 0.4711773326819736, 0.47166585246702486, 0.47215437225207624, 0.4726428920371275, 0.47313141182217877, 0.47361993160723004, 0.4741084513922813, 0.4745969711773327, 0.47508549096238395, 0.4755740107474352, 0.4760625305324866, 0.47655105031753786, 0.4770395701025891, 0.4775280898876404, 0.47801660967269166, 0.47850512945774304, 0.4789936492427943, 0.4794821690278456, 0.47997068881289695, 0.4804592085979482, 0.4809477283829995, 0.48143624816805075, 0.481924767953102, 0.4824132877381534, 0.48290180752320466, 0.48339032730825593, 0.4838788470933073, 0.4843673668783586, 0.48485588666340984, 0.4853444064484611, 0.4858329262335124, 0.48632144601856375, 0.486809965803615, 0.4872984855886663, 0.48778700537371766, 0.48827552515876893, 0.4887640449438202, 0.48925256472887146, 0.48974108451392273, 0.4902296042989741, 0.4907181240840254, 0.49120664386907664, 0.491695163654128, 0.4921836834391793, 0.49267220322423055, 0.4931607230092818, 0.4936492427943331, 0.49413776257938447, 0.49462628236443573, 0.495114802149487, 0.4956033219345384, 0.49609184171958964, 0.4965803615046409, 0.4970688812896922, 0.49755740107474344, 0.4980459208597948, 0.4985344406448461, 0.49902296042989736, 0.49951148021494873, 0.5]
  out "X size (V)":dbl=20.0
  out "Y size (V)":dbl=10.0
  out "Eanable COM":bool
  out "Machine ID":string
  out "Image bits":u8=16
  out "FI scaling":u8=1
  out "X aln":sgl
  out "Y aln":sgl
  out "Mag":dbl=5582.6
  out "Screen pixel factor":dbl=0.25
  # "Hz"
  # "Scanning time"
  # "m"
  # "s"
  # "Det"
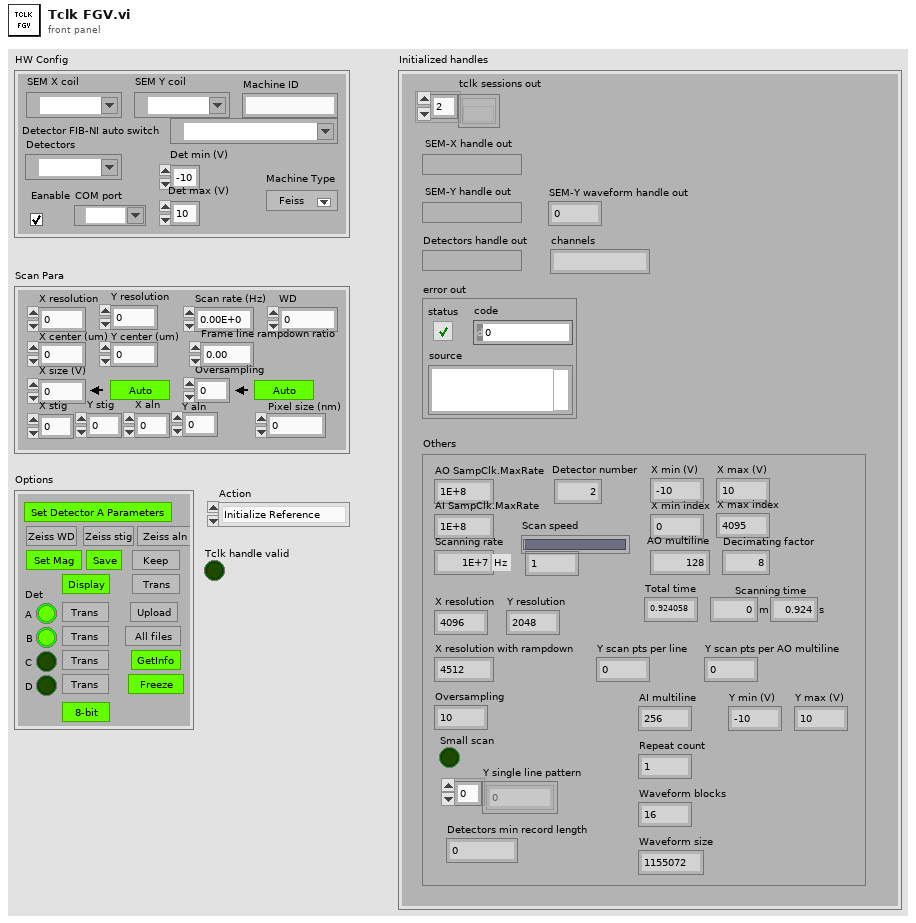
[diagram p1: front panel]
types:
  T1 = enum16{"Initialize Reference", "Get Reference", "Close Reference"}
  T2 = cluster{"sessions out":refnum<k20>[], "SEM-X handle out":refnum<k15>, "SEM-Y handle out":refnum<k15>, "SEM-Y waveform handle out":i32, "Detectors handle out":refnum<k15>, "channels":string, "error out":errorcluster, "Others":cluster{"AO SampClk.MaxRate":dbl, "AI SampClk.MaxRate":dbl, "AO rate":dbl, "Scan speed":u8, "Detector number":u8, "X min (V)":dbl, "X max (V)":dbl, "X min index":i32, "X max index":i32, "Y min (V)":dbl, "Y max (V)":dbl, "AO multiline":u32, "Decimating factor":u16, "Total time":dbl, "Scan time (m)":dbl, "Scan time (s)":dbl, "X resolution":u32, "Y resolution":u32, "X resolution with rampdown":i32, "Oversampling":u32, "Y scan pts per line":i32, "Y scan pts per AO multiline":i32, "Small scan":bool, "Y single line pattern":dbl[], "Detectors min record length":u32, "Waveform blocks":u32, "Repeat count":u32, "Waveform size":u32, "AI multiline":u16}}
  T3 = cluster{"X resolution":u32, "Y resolution":u32, "X center (um)":dbl, "Y center (um)":dbl, "X size (V)":dbl, "X size auto":bool, "X stig":sgl, "Y stig":sgl, "X aln":sgl, "Y aln":sgl, "Scan rate (Hz)":u32, "Oversampling":u32, "Oversampling auto":bool, "Frame line rampdown ratio":sgl, "Pixel size (nm)":sgl, "WD":sgl}
  T4 = cluster{"SEM X coil":refnum<k15>, "SEM Y coil":refnum<k15>, "Detectors":refnum<k15>, "Det min (V)":dbl, "Det max (V)":dbl, "Eanable COM":bool, "COM port":refnum<visa-resource-name>, "Detector FIB-NI auto switch":tag, "Machine Type":u8, "Machine ID":string}
  T5 = cluster{"GetInfo":bool, "Set Det A para":bool, "Set WD":bool, "Set Mag":bool, "Set stig":bool, "Set aln":bool, "Display":bool, "Save":bool, "8-bit":bool, "Detector A":bool, "Detector B":bool, "Detector C":bool, "Detector D":bool, "Inverse A":bool, "Inverse B":bool, "Inverse C":bool, "Inverse D":bool, "Inverse PNG":bool, "Freeze":bool, "PNG only":bool, "Upload":bool, "Delete after upload":bool}
  T6 = cluster{"SEM X coil":refnum<k15>, "SEM Y coil":refnum<k15>, "Detectors":refnum<k15>, "Det min (V)":sgl, "Det max (V)":sgl, "X resolution":u32, "Y resolution":u32, "X size (V)":sgl, "Scan rate (Hz)":u32, "Oversampling":u32, "Frame line rampdown ratio":sgl, "Pixel size (nm)":sgl, "Detector A":bool, "Detector B":bool, "Detector C":bool, "Detector D":bool}
  T7 = typedef "niFgen Output Mode.ctl" = u32
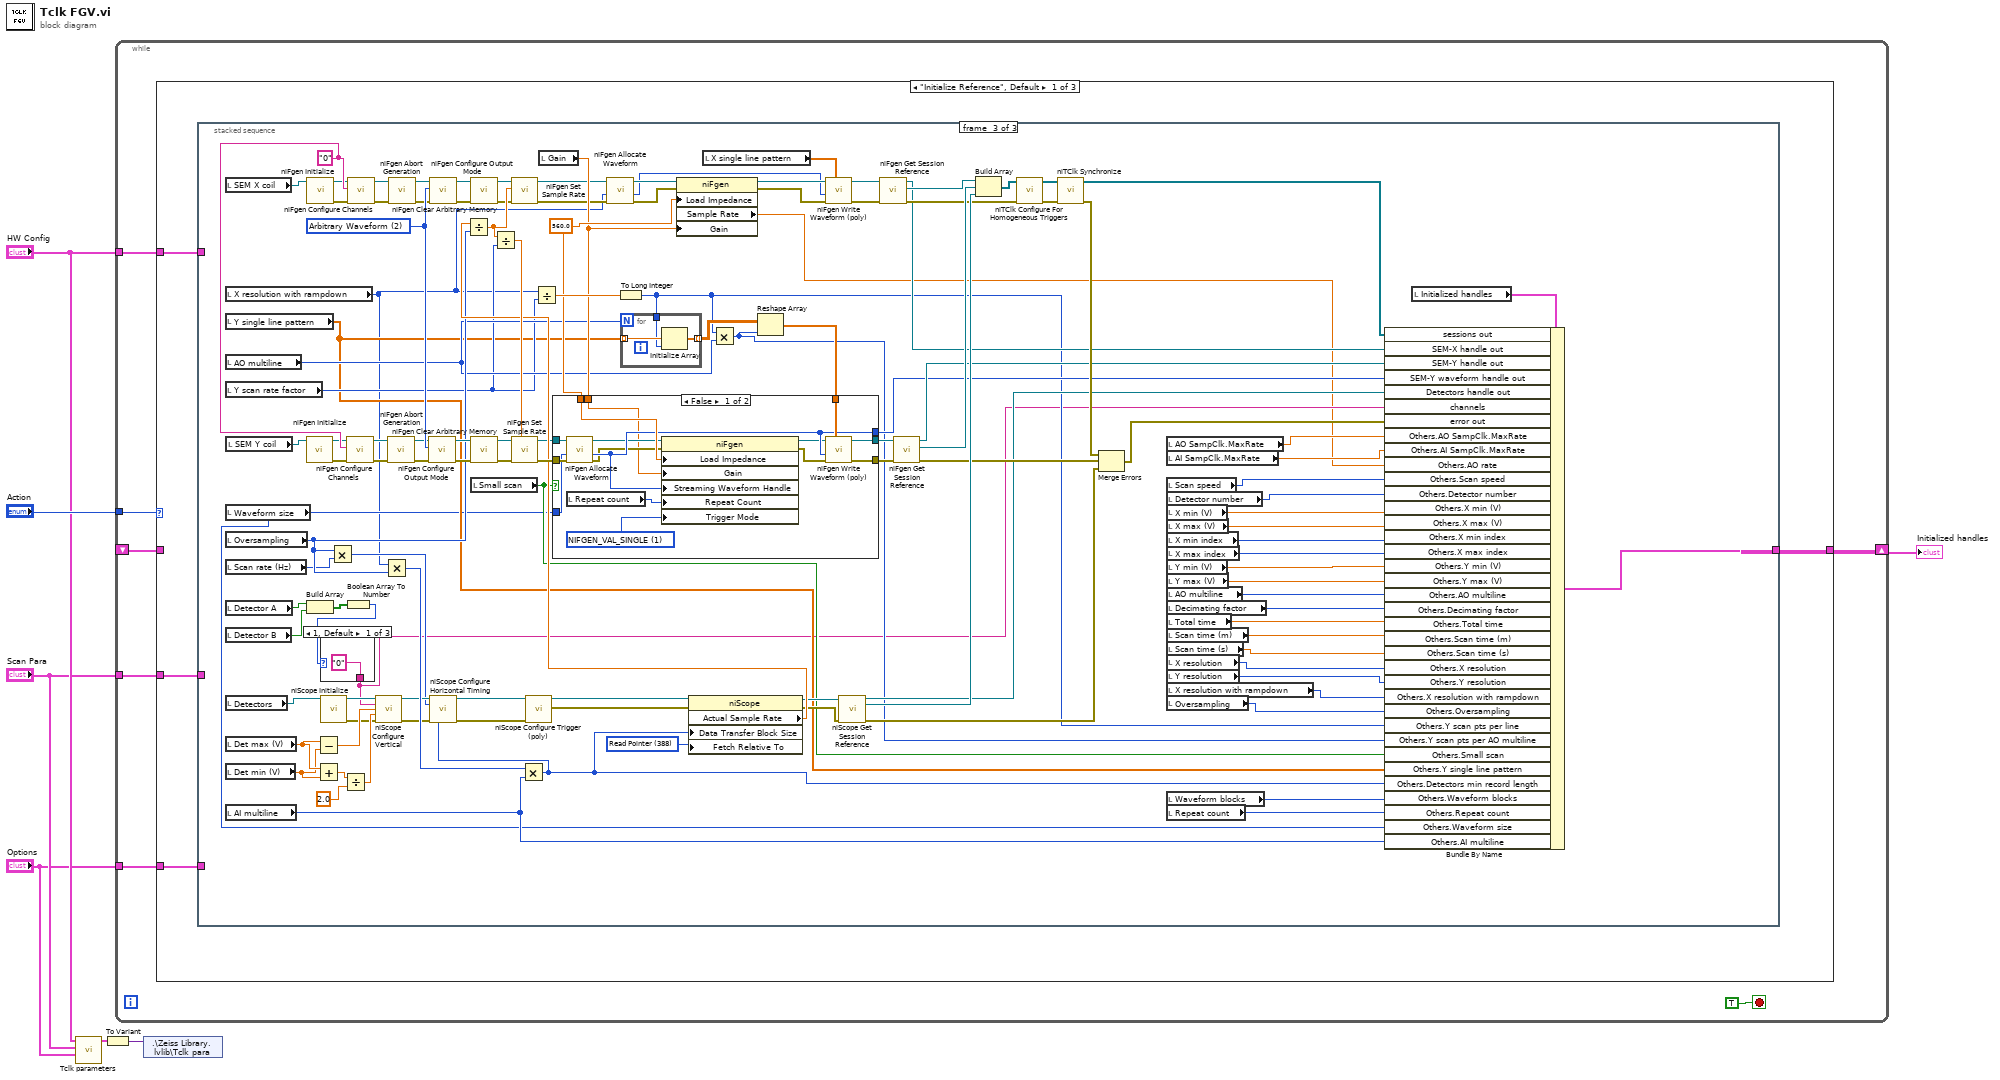
[diagram p0: block diagram]
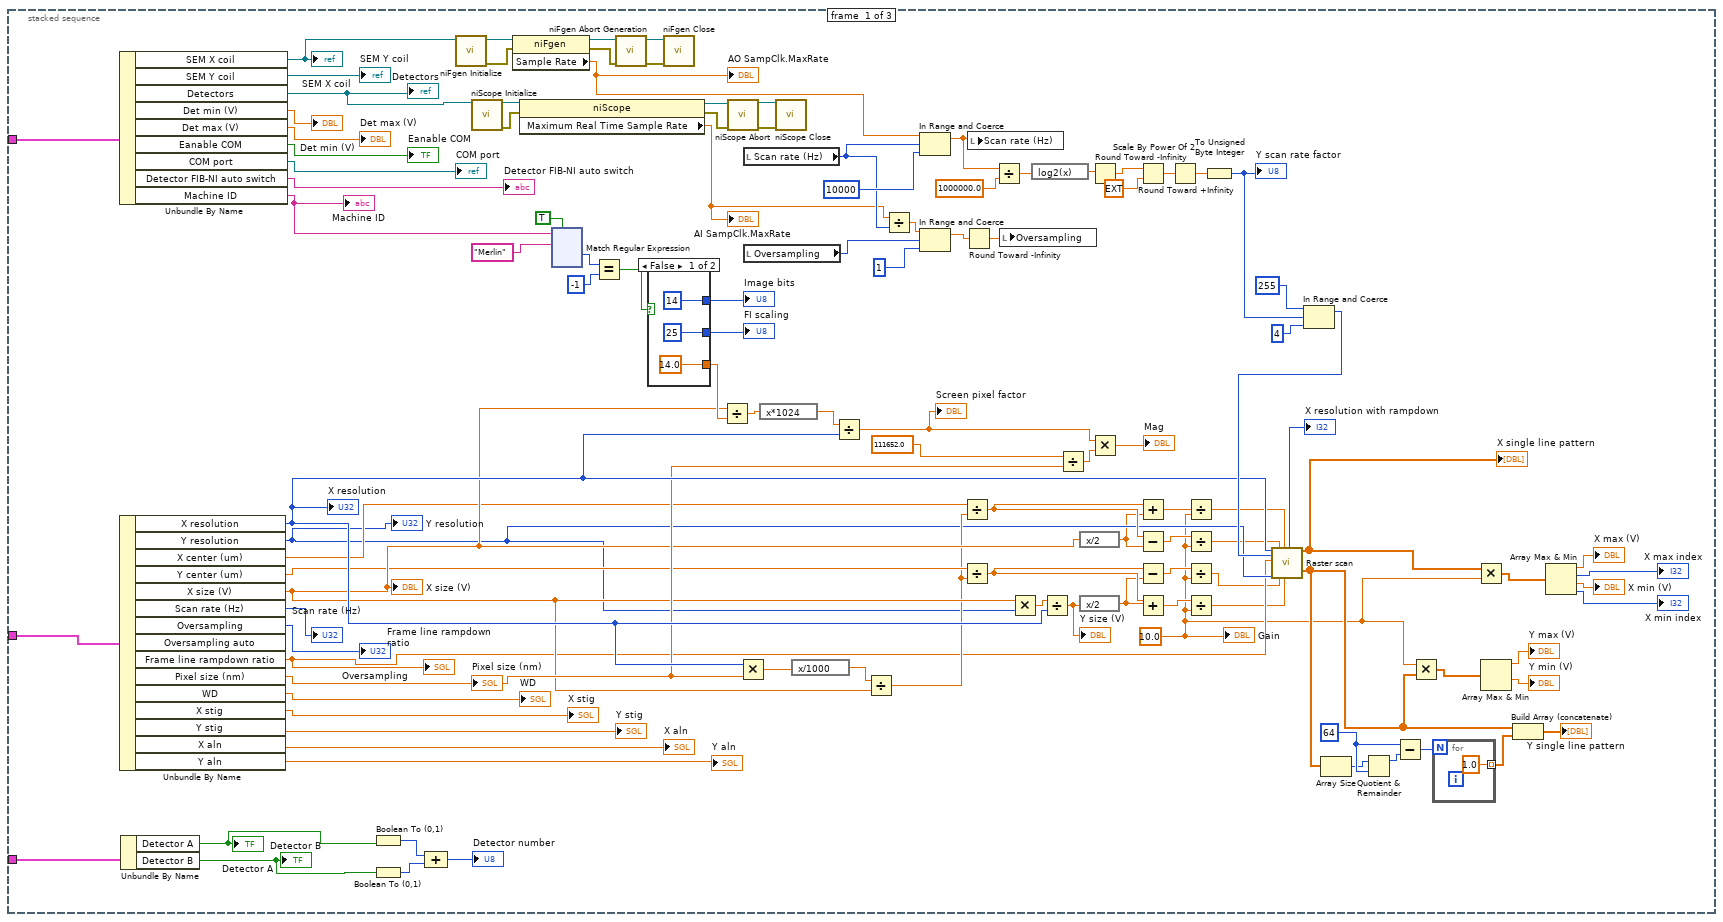
[diagram p2: hidden frame]
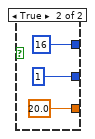
[diagram p3: hidden frame]
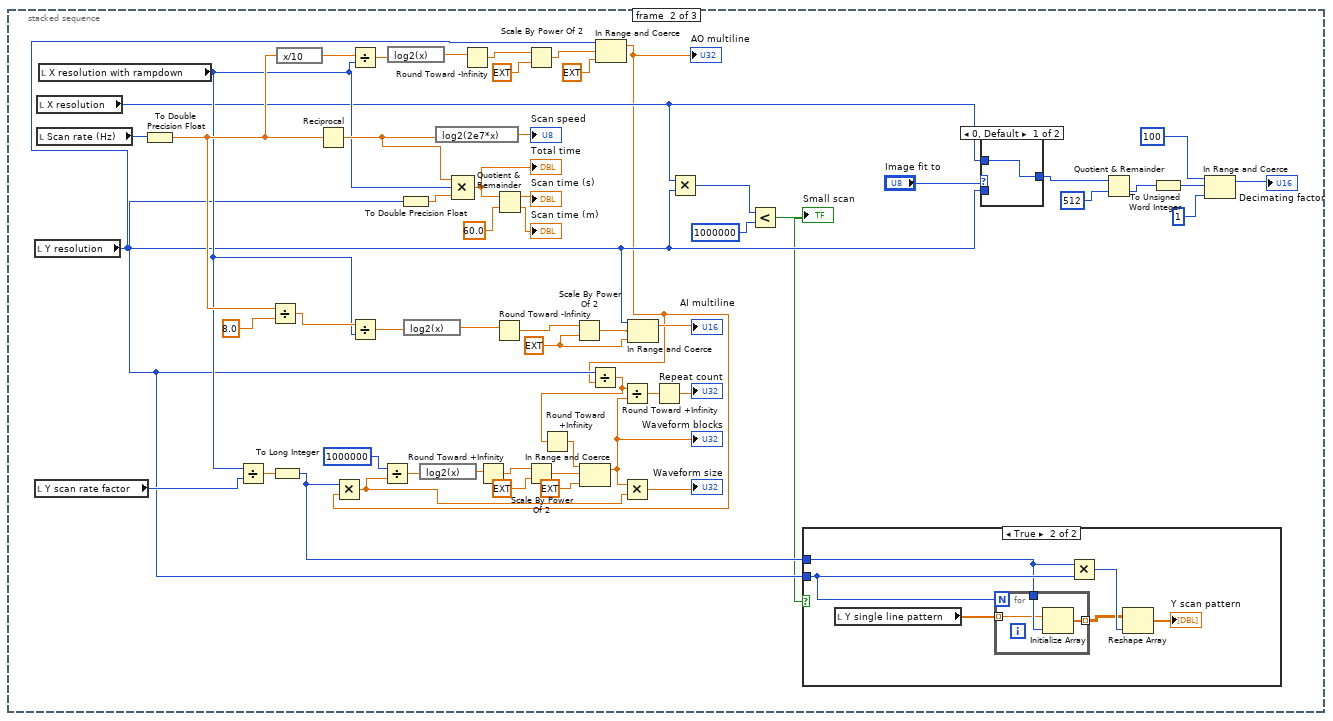
[diagram p4: hidden frame]
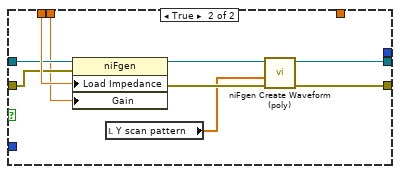
[diagram p7: hidden frame]
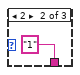
[diagram p8: hidden frame]
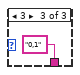
[diagram p9: hidden frame]
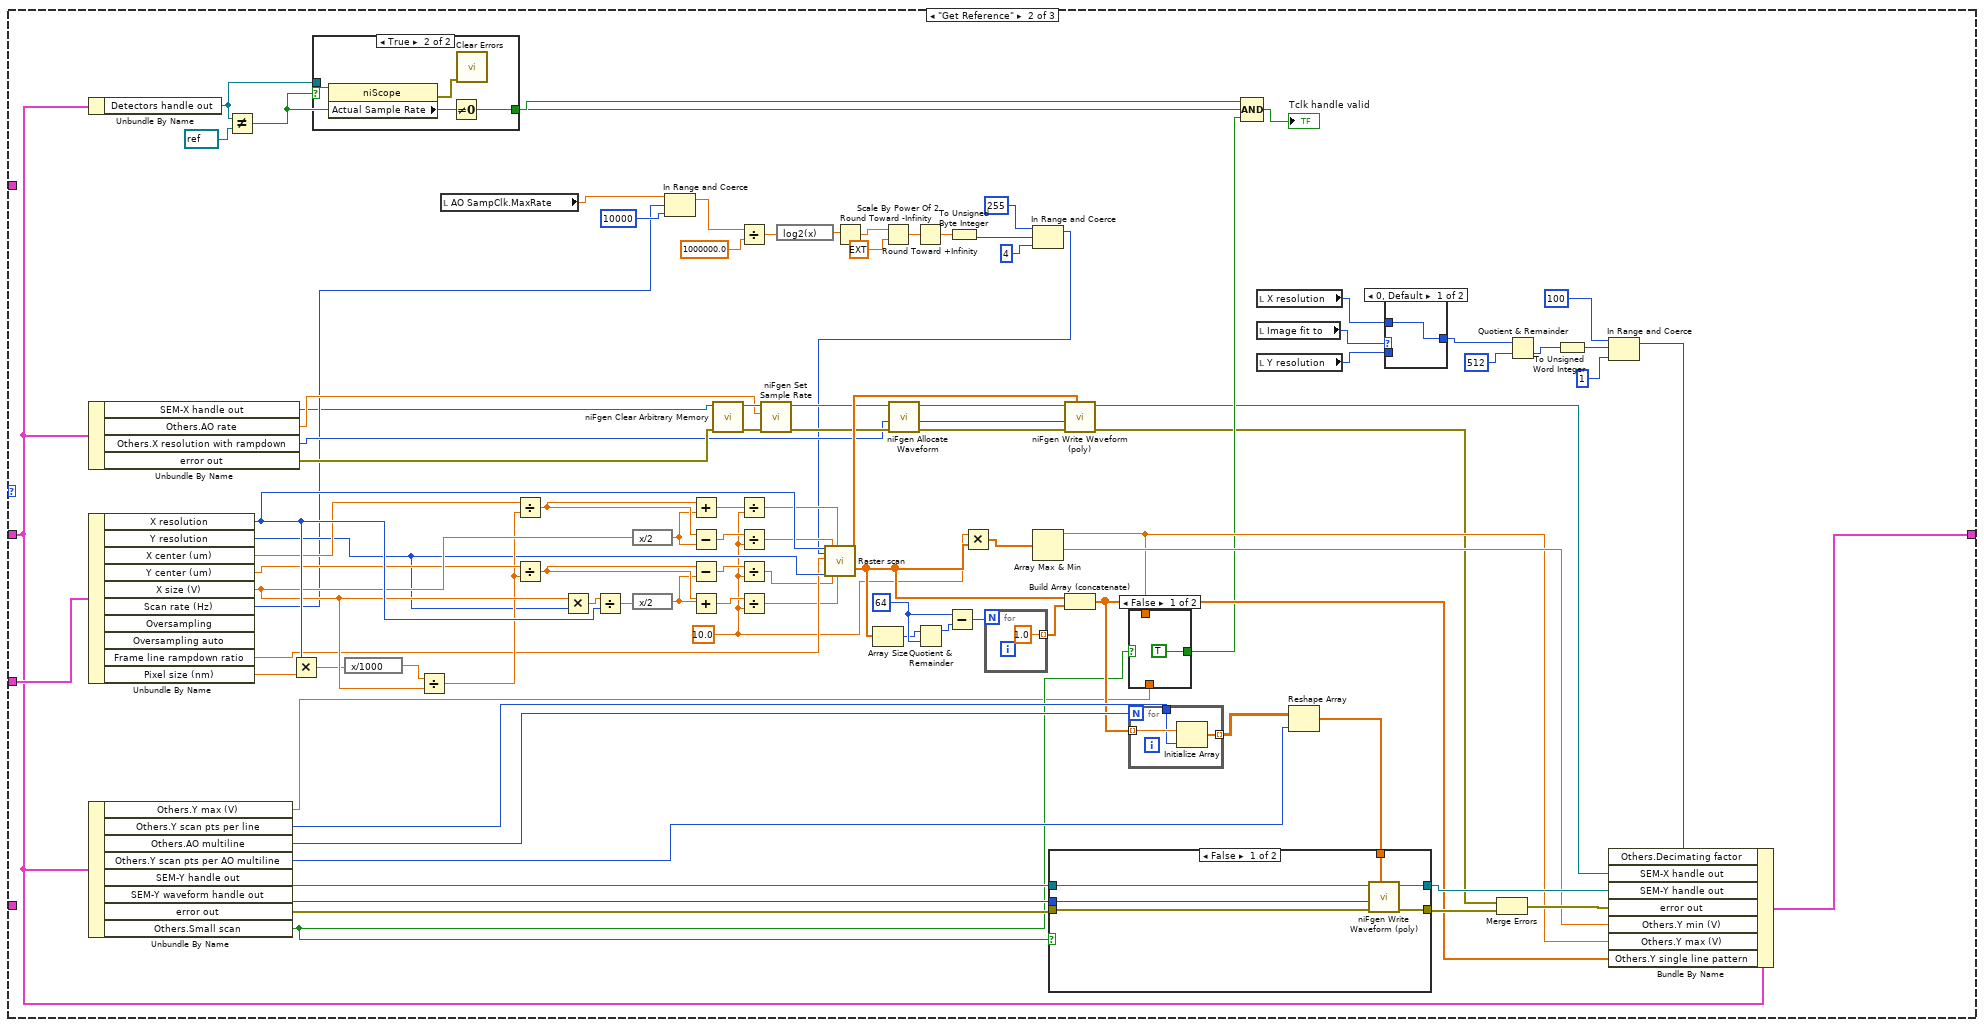
[diagram p10: hidden frame]
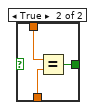
[diagram p12: hidden frame]
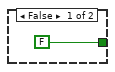
[diagram p13: hidden frame]
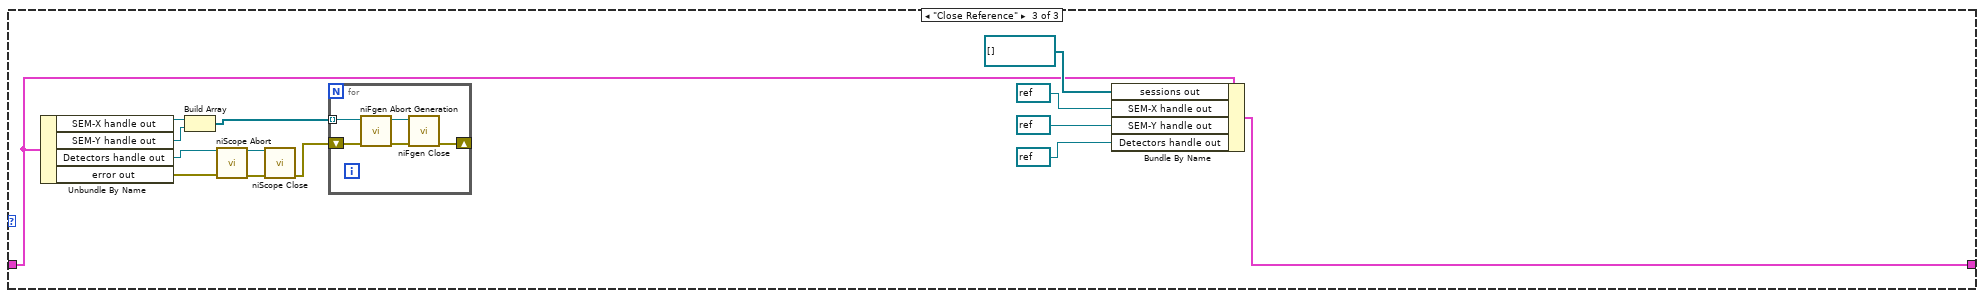
[diagram p15: hidden frame]
diagram:
  n1 = call "Tclk parameters.vi"("Options"="Options", "Scan Para"="Scan Para", "HW Config"="HW Config") -> ("Tclk para out"=w1:T6)  [unwired: 7 in, 1 out]
  n2 = To Variant(anything=w1) -> (Variant=w5:variant)
  n3 = while {
    shift-right: [w13] -> w7
    shift-left: _ -> [w12]
    tunnel: "Action" -> [w11]
    tunnel: "HW Config" -> [w10]
    tunnel: "Scan Para" -> [w9]
    tunnel: "Options" -> [w8]
    stop <- TRUE stop-if-true
    n4 = case shown="\"Initialize Reference\", Default" w11 {
      tunnel: [w18 w565 w598] -> w13
      tunnel: w12 -> [_ w524 w597]
      tunnel: w10 -> [w17 _ _]
      tunnel: w9 -> [w16 w527 _]
      tunnel: w8 -> [w15 _ _]
      frame "Initialize Reference", Default {
        n5 = stacked-sequence {
          tunnel: [_ _ w359] -> w18
          tunnel: w17 -> [w37 _ _]
          tunnel: w16 -> [w36 _ _]
          tunnel: w15 -> [w35 _ _]
          frame #0 {
            w130 = 64 ("y")
            w20 = 10.0 ("x")
            n6 = Unbundle By Name(w37) -> ("SEM X coil"=w74:refnum<k15>, "SEM Y coil"=→"SEM Y coil":refnum<k15>, "Detectors"=w71:refnum<k15>, "Det min (V)"=→"Det min (V)":dbl, "Det max (V)"=→"Det max (V)":dbl, "Eanable COM"=→"Eanable COM":bool, "COM port"=→"COM port":refnum<visa-resource-name>, "Detector FIB-NI auto switch"=→"Detector FIB-NI auto switch":tag, "Machine ID"=w109:string)
            "SEM X coil" <- w74
            "Detectors" <- w71
            "Machine ID" <- w109
            n7 = Unbundle By Name(w36) -> ("X resolution"=w121:u32, "Y resolution"=w86:u32, "X center (um)"=w101:dbl, "Y center (um)"=w103:dbl, "X size (V)"=w118:dbl, "Scan rate (Hz)"=→"Scan rate (Hz)":u32, "Oversampling"=→"Oversampling":u32, "Frame line rampdown ratio"=w67:sgl, "Pixel size (nm)"=w120:sgl, "WD"=→"WD":sgl, "X stig"=→"X stig":sgl, "Y stig"=→"Y stig":sgl, "X aln"=→"X aln":sgl, "Y aln"=→"Y aln":sgl)  [unwired: 1 out]
            "X resolution" <- w121
            "Y resolution" <- w86
            "Frame line rampdown ratio" <- w67
            "Pixel size (nm)" <- w120
            "X size (V)" <- w118
            n8 = Unbundle By Name(w35) -> ("Detector A"=w26:bool, "Detector B"=w25:bool)
            "Detector A" <- w26
            "Detector B" <- w25
            n9 = Boolean To (0,1)(Boolean=w26) -> (0, 1=w28:i16)
            n10 = Boolean To (0,1)(Boolean=w25) -> (0, 1=w29:i16)
            n11 = Compound Arithmetic op=ADD(w28, w29) -> (→"Detector number":i16)
            n12 = call <instrlib>:"niFgen Initialize.vi"("Resource Name"=w74) -> ("error out"=w84:errorcluster, "Instrument Handle Out"=w73:refnum<k15>)  [unwired: 9 in]
            n13 = call <instrlib>:"niScope Initialize.vi"("resource name"=w71) -> ("instrument handle"=w72:refnum<k15>, "error out"=w78:errorcluster)  [unwired: 13 in]
            n14 = property class="niFgen"(reference=w73, error in=w84) -> (reference out=w82:refnum<k15>, error out=w83:errorcluster, "Sample Rate"=w39:dbl)
            "AO SampClk.MaxRate" <- w39
            n15 = property class="niScope"(reference=w72, error in=w78) -> (reference out=w77:refnum<k15>, error out=w79:errorcluster, "Maximum Real Time Sample Rate"=w38:dbl)
            "AI SampClk.MaxRate" <- w38
            n16 = xnode "Match Regular Expression"("input string"=w109, "regular expression"="Merlin", "ignore case? (F)"=TRUE) -> ("offset past match"=w107:i32)  [unwired: 3 in, 4 out]
            n17 = Equal?(x=w107, y=-1) -> (x = y?=w111:bool)
            n18 = call <instrlib>:"niFgen Abort Generation.vi"("error in (no error)"=w83, "Instrument Handle"=w82) -> ("error out"=w80:errorcluster, "Instrument Handle Out"=w81:refnum<k15>)  [unwired: 8 in]
            n19 = case shown="False" w111 {
              tunnel: [u8 14 ("t") u8 16 ("t")] -> w110
              tunnel: [u8 25 ("t") u8 1 ("t")] -> w112
              tunnel: [14.0 ("y") 20.0 ("y")] -> w119
              frame False {
              }
              frame True {
              }
            }
            "Image bits" <- w110
            "FI scaling" <- w112
            n20 = call <instrlib>:"niFgen Close.vi"("error in (no error)"=w80, "Instrument Handle"=w81) -> ()  [unwired: 9 in, 1 out]
            n21 = Divide(x=w118, y=w119) -> (x/y=w115:dbl)
            n22 = call <instrlib>:"niScope Abort.vi"("instrument handle"=w77, "error in"=w79) -> ("instrument handle out"=w75:refnum<k15>, "error out"=w76:errorcluster)  [unwired: 12 in]
            n23 = Multiply(x=w121, y=w120) -> (x*y=w98:sgl)
            n24 = local read "Scan rate (Hz)"() -> (w40:u32)
            n25 = local read "Oversampling"() -> (w43:u32)
            n26 = expression code="x*1024"(w115) -> (w123:dbl)
            n27 = call <instrlib>:"niScope Close.vi"("instrument handle"=w75, "error in"=w76) -> ()  [unwired: 13 in, 1 out]
            n28 = expression code="x/1000"(w98) -> (w99:sgl)
            n29 = Divide(x=w123, y=w121) -> (x/y=w124:dbl)
            "Screen pixel factor" <- w124
            n30 = Divide(x=w99, y=w118) -> (x/y=w102:dbl)
            n31 = Divide(x=w38, y=w40) -> (x/y=w45:dbl)
            n32 = In Range and Coerce(upper limit=w39, x=w40, lower limit=u32 10000) -> (coerced(x)=w88:dbl)  [unwired: 1 out]
            n33 = In Range and Coerce(upper limit=w45, x=w43, lower limit=u8 1) -> (coerced(x)=w44:dbl)  [unwired: 1 out]
            n34 = Divide(x=w101, y=w102) -> (x/y=w100:dbl)
            n35 = Divide(x=w103, y=w102) -> (x/y=w104:dbl)
            n36 = Round Toward -Infinity(1:w44) -> (0:w41:dbl)
            n37 = local write "Scan rate (Hz)"(w88) -> ()
            n38 = Divide(x=w88, y=1000000.0) -> (x/y=w93:dbl)
            n39 = local write "Oversampling"(w41) -> ()
            n40 = Multiply(x=w118, y=w86) -> (x*y=w85:dbl)
            n41 = expression code="log2(x)"(w93) -> (w91:dbl)
            n42 = Divide(x=w85, y=w121) -> (x/y=w87:dbl)
            "Y size (V)" <- w87
            n43 = Divide(x=111652.0, y=w120) -> (x/y=w117:dbl)
            n44 = expression code="x/2"(w118) -> (w58:dbl)
            n45 = expression code="x/2"(w87) -> (w57:dbl)
            n46 = Round Toward -Infinity(1:w91) -> (0:w92:dbl)
            n47 = Multiply(x=w124, y=w117) -> (x*y=→"Mag":dbl)
            n48 = Scale By Power Of 2(n=w92, x=ext 1.0) -> (x*2^n=w94:ext)
            n49 = Add(x=w100, y=w58) -> (x+y=w60:dbl)
            n50 = Subtract(x=w100, y=w58) -> (x-y=w59:dbl)
            n51 = Subtract(x=w104, y=w57) -> (x-y=w61:dbl)
            n52 = Add(x=w104, y=w57) -> (x+y=w62:dbl)
            n53 = Round Toward +Infinity(x=w94) -> (ceil(x): smallest int >= x=w95:ext)
            n54 = Divide(x=w60, y=w20) -> (x/y=w64:dbl)
            n55 = Divide(x=w59, y=w20) -> (x/y=w63:dbl)
            n56 = Divide(x=w61, y=w20) -> (x/y=w65:dbl)
            n57 = Divide(x=w62, y=w20) -> (x/y=w66:dbl)
            n58 = To Unsigned Byte Integer(number=w95) -> (unsigned 8bit integer=w96:u8)
            "Y scan rate factor" <- w96
            n59 = In Range and Coerce(upper limit=u8 255 ("X round to"), x=w96, lower limit=u8 4 ("X round to")) -> (coerced(x)=w125:u8)  [unwired: 1 out]
            n60 = call "Raster scan.vi"("X resolution"=w121, "X round to"=w125, "Frame line rampdown ratio"=w67, "Y resolution"=w86, "X start"=w63, "Y start"=w65, "X end"=w64, "Y end"=w66) -> ("X resolution with rampdown"=→"X resolution with rampdown":i32, "X single line pattern"=w19:dbl[], "Y single line pattern"=w21:dbl[])  [unwired: 4 in, 5 out]
            "X single line pattern" <- w19
            n61 = Array Size(array=w21) -> (size(s)=w126:i32)
            n62 = Quotient & Remainder(x=w126, y=w130) -> (x-y*floor(x/y)=w131:i32)  [unwired: 1 out]
            n63 = Subtract(x=w130, y=w131) -> (x-y=w129:i32)
            n64 = Multiply(x=w20, y=w21) -> (x*y=w22:dbl[])
            n65 = for {
              N: w129 -> [_]
              tunnel: [1.0 ("x")] -> w127 mode=indexing
            }
            n66 = Multiply(x=w19, y=w20) -> (x*y=w34:dbl[])
            n67 = Array Max & Min(array=w22) -> (max value=→"Y max (V)":dbl, min value=→"Y min (V)":dbl)  [unwired: 2 out]
            n68 = Build Array (concatenate)(w21, w127) -> (→"Y single line pattern":dbl[])
            n69 = Array Max & Min(array=w34) -> (max value=→"X max (V)":dbl, max index (indices)=→"X max index":i32, min value=→"X min (V)":dbl, min index (indices)=→"X min index":i32)
            "Gain" <- w20
          }
          frame #1 {
            w286 = ext 1.0 ("x")
            n70 = local read "Y resolution"() -> (w257:u32)
            n71 = local read "Y scan rate factor"() -> (w267:u8)
            n72 = local read "X resolution"() -> (w258:u32)
            n73 = local read "Scan rate (Hz)"() -> (w268:u32)
            n74 = local read "X resolution with rampdown"() -> (w269:i32)
            n75 = To Double Precision Float(number=w268) -> (double precision float=w304:dbl)
            n76 = Divide(x=w269, y=w267) -> (x/y=w287:dbl)
            n77 = Divide(x=w304, y=8.0) -> (x/y=w279:dbl)
            n78 = To Long Integer(number=w287) -> (32bit integer=w266:i32)
            n79 = expression code="x/10"(w304) -> (w305:dbl)
            n80 = Reciprocal(x=w304) -> (1/x=w276:dbl)
            n81 = Divide(x=w305, y=w269) -> (x/y=w274:dbl)
            n82 = Divide(x=w279, y=w269) -> (x/y=w283:dbl)
            n83 = expression code="log2(x)"(w274) -> (w273:dbl)
            n84 = To Double Precision Float(number=w257) -> (double precision float=w275:dbl)
            n85 = expression code="log2(x)"(w283) -> (w281:dbl)
            n86 = expression code="log2(2e7*x)"(w276) -> (→"Scan speed":dbl)
            n87 = Compound Arithmetic op=MULTIPLY(w276, w269, w275) -> (w253:dbl)
            "Total time" <- w253
            n88 = Round Toward -Infinity(1:w273) -> (0:w270:dbl)
            n89 = Round Toward -Infinity(1:w281) -> (0:w282:dbl)
            n90 = Quotient & Remainder(x=w253, y=60.0) -> (x-y*floor(x/y)=→"Scan time (s)":dbl, floor(x/y)=→"Scan time (m)":dbl)
            n91 = Scale By Power Of 2(n=w270, x=ext 1.0) -> (x*2^n=w272:ext)
            n92 = Scale By Power Of 2(n=w282, x=w286) -> (x*2^n=w285:ext)
            n93 = In Range and Coerce(upper limit=w257, x=w272, lower limit=ext 64.0 ("x")) -> (coerced(x)=w255:ext)  [unwired: 1 out]
            "AO multiline" <- w255
            n94 = Multiply(x=w266, y=w255) -> (x*y=w294:ext)
            n95 = Divide(x=u32 1000000, y=w294) -> (x/y=w291:ext)
            n96 = expression code="log2(x)"(w291) -> (w293:ext)
            n97 = Round Toward +Infinity(x=w293) -> (ceil(x): smallest int >= x=w292:ext)
            n98 = Scale By Power Of 2(n=w292, x=ext 1.0) -> (x*2^n=w297:ext)
            n99 = Divide(x=w257, y=w255) -> (x/y=w299:ext)
            n100 = Round Toward +Infinity(x=w299) -> (ceil(x): smallest int >= x=w300:ext)
            n101 = In Range and Coerce(upper limit=w300, x=w297, lower limit=ext 2.0) -> (coerced(x)=w296:ext)  [unwired: 1 out]
            "Waveform blocks" <- w296
            n102 = Divide(x=w299, y=w296) -> (x/y=w288:ext)
            n103 = Multiply(x=w296, y=w294) -> (x*y=→"Waveform size":ext)
            n104 = In Range and Coerce(upper limit=w257, x=w285, lower limit=w286) -> (coerced(x)=→"AI multiline":ext)  [unwired: 1 out]
            n105 = Round Toward +Infinity(x=w288) -> (ceil(x): smallest int >= x=→"Repeat count":ext)
            n106 = Multiply(x=w258, y=w257) -> (x*y=w302:u32)
            n107 = Less?(x=w302, y=u32 1000000) -> (x < y?=w256:bool)
            "Small scan" <- w256
            n108 = case shown="True" w256 {
              tunnel: w266 -> [_ w308]
              tunnel: w257 -> [_ w309]
              frame False {
              }
              frame True {
                n109 = local read "Y single line pattern"() -> (w311:dbl[])
                n110 = for {
                  N: w309 -> [_]
                  tunnel: [w316] -> w312 mode=indexing
                  tunnel: w308 -> [w315]
                  tunnel: w311 -> [w314] mode=indexing
                  n111 = Initialize Array(w314, w315) -> (w316:dbl[])
                }
                n112 = Multiply(x=w308, y=w309) -> (x*y=w313:u32)
                n113 = Reshape Array(w312, w313) -> (→"Y scan pattern":dbl[])
              }
            }
            n114 = case shown="0, Default" "Image fit to" {
              tunnel: w258 -> [w306 _]
              tunnel: w257 -> [_ w307]
              tunnel: [w306 w307] -> w262
              frame 0, Default {
              }
              frame 1 {
              }
            }
            n115 = Quotient & Remainder(x=w262, y=u32 512) -> (floor(x/y)=w264:u32)  [unwired: 1 out]
            n116 = To Unsigned Word Integer(number=w264) -> (unsigned 16bit integer=w259:u16)
            n117 = In Range and Coerce(upper limit=u16 100, x=w259, lower limit=u16 1) -> (coerced(x)=→"Decimating factor":u16)  [unwired: 1 out]
          }
          frame #2 {
            w421 = 560.0 ("Output:Load Impedance")
            w432 = 388 items=["Start"=482, "Trigger"=483, "Pretrigger"=477, "Now"=481, "Read Pointer"=388] ("Fetch:Fetch Relative To")
            w402 = T7 2 items=["Standard Function", "Frequency List", "Arbitrary Waveform", "Arbitrary Sequence", "Script"] ("Output Mode")
            w425 = "0" ("Channels")
            n118 = local read "SEM X coil"() -> (w384:refnum<k15>)
            n119 = local read "X resolution with rampdown"() -> (w319:i32)
            n120 = local read "Y single line pattern"() -> (w352:dbl[])
            n121 = local read "AO multiline"() -> (w376:u32)
            n122 = local read "Y scan rate factor"() -> (w375:u8)
            n123 = local read "Waveform size"() -> (w349:u32)
            n124 = local read "Oversampling"() -> (w381:u32)
            n125 = local read "Scan rate (Hz)"() -> (w380:u32)
            n126 = local read "Detector A"() -> (w374:bool)
            n127 = local read "Detector B"() -> (w373:bool)
            n128 = local read "Detectors"() -> (w379:refnum<k15>)
            n129 = local read "Det max (V)"() -> (w378:dbl)
            n130 = local read "Det min (V)"() -> (w377:dbl)
            n131 = local read "AI multiline"() -> (w350:u16)
            n132 = local read "SEM Y coil"() -> (w382:refnum<k15>)
            n133 = call <instrlib>:"niFgen Initialize.vi"("Resource Name"=w382) -> ("error out"=w394:errorcluster, "Instrument Handle Out"=w397:refnum<k15>)  [unwired: 9 in]
            n134 = call <instrlib>:"niFgen Initialize.vi"("Resource Name"=w384) -> ("error out"=w392:errorcluster, "Instrument Handle Out"=w389:refnum<k15>)  [unwired: 9 in]
            n135 = Build Array(w374, w373) -> (w433:bool[])
            n136 = Subtract(x=w378, y=w377) -> (x-y=w416:dbl)
            n137 = Add(x=w378, y=w377) -> (x+y=w417:dbl)
            n138 = call <instrlib>:"niScope Initialize.vi"("resource name"=w379) -> ("instrument handle"=w407:refnum<k15>, "error out"=w408:errorcluster)  [unwired: 13 in]
            n139 = Multiply(x=w381, y=w380) -> (x*y=w420:u32)
            n140 = Divide(x=w417, y=2.0) -> (x/y=w419:dbl)
            n141 = Boolean Array To Number(Boolean array=w433) -> (number=w434:u32)
            n142 = case shown="1, Default" w434 {
              tunnel: ["0" ("channels") "1" ("channels") "0,1" ("channels")] -> w346
              frame 1, Default {
              }
              frame 2 {
              }
              frame 3 {
              }
            }
            n143 = call <instrlib>:"niFgen Configure Channels.vi"("error in (no error)"=w394, "Channels"=w425, "Instrument Handle"=w397) -> ("error out"=w395:errorcluster, "Instrument Handle Out"=w396:refnum<k15>)  [unwired: 7 in]
            n144 = call <instrlib>:"niFgen Configure Channels.vi"("error in (no error)"=w392, "Channels"=w425, "Instrument Handle"=w389) -> ("error out"=w391:errorcluster, "Instrument Handle Out"=w390:refnum<k15>)  [unwired: 7 in]
            n145 = call <instrlib>:"niScope Configure Vertical.vi"("instrument handle"=w407, "channels"=w346, "vertical range"=w416, "vertical offset"=w419, "error in"=w408) -> ("instrument handle out"=w436:refnum<k15>, "error out"=w409:errorcluster)  [unwired: 9 in]
            n146 = Multiply(x=w319, y=w381) -> (x*y=w437:u32)
            n147 = call <instrlib>:"niFgen Abort Generation.vi"("error in (no error)"=w395, "Instrument Handle"=w396) -> ("error out"=w398:errorcluster, "Instrument Handle Out"=w399:refnum<k15>)  [unwired: 8 in]
            n148 = call <instrlib>:"niFgen Abort Generation.vi"("error in (no error)"=w391, "Instrument Handle"=w390) -> ("error out"=w388:errorcluster, "Instrument Handle Out"=w387:refnum<k15>)  [unwired: 8 in]
            n149 = call <instrlib>:"niFgen Configure Output Mode.vi"("error in (no error)"=w398, "Output Mode (default: 0=Standard Function)"=w402, "Instrument Handle"=w399) -> ("error out"=w401:errorcluster, "Instrument Handle Out"=w400:refnum<k15>)  [unwired: 6 in]
            n150 = call <instrlib>:"niFgen Configure Output Mode.vi"("error in (no error)"=w388, "Output Mode (default: 0=Standard Function)"=w402, "Instrument Handle"=w387) -> ("error out"=w385:errorcluster, "Instrument Handle Out"=w386:refnum<k15>)  [unwired: 6 in]
            n151 = call <instrlib>:"niFgen Clear Arbitrary Memory.vi"("error in (no error)"=w385, "Instrument Handle"=w386) -> ("error out"=w404:errorcluster, "Instrument Handle Out"=w403:refnum<k15>)  [unwired: 8 in]
            n152 = call <instrlib>:"niFgen Clear Arbitrary Memory.vi"("error in (no error)"=w401, "Instrument Handle"=w400) -> ("error out"=w406:errorcluster, "Instrument Handle Out"=w405:refnum<k15>)  [unwired: 8 in]
            n153 = local read "Small scan"() -> (w353:bool)
            n154 = Multiply(x=w437, y=w350) -> (x*y=w351:u32)
            n155 = call <instrlib>:"niScope Configure Horizontal Timing.vi"("instrument handle"=w436, "min sample rate"=w420, "error in"=w409, "min record length"=w351) -> ("instrument handle out"=w410:refnum<k15>, "error out"=w411:errorcluster)  [unwired: 10 in]
            n156 = call-poly <instrlib>:"niScope Configure Trigger (poly).vi"("instrument handle"=w410, "error in"=w411) -> ("instrument handle out"=w412:refnum<k15>, "error out"=w414:errorcluster)  [unwired: 12 in]
            n157 = Divide(x=w319, y=w375) -> (x/y=w431:dbl)
            n158 = local read "Gain"() -> (w383:dbl)
            n159 = To Long Integer(number=w431) -> (32bit integer=w355:i32)
            n160 = for {
              N: w376 -> [_]
              tunnel: w352 -> [w469] mode=indexing
              tunnel: [w468] -> w426 mode=indexing
              tunnel: w355 -> [w467]
              n161 = Initialize Array(w469, w467) -> (w468:dbl[])
            }
            n162 = property class="niScope"(reference=w412, error in=w414, "Data Transfer Block Size"=w351, "Fetch Relative To"=w432) -> (reference out=w413:refnum<k15>, error out=w415:errorcluster, "Actual Sample Rate"=w422:dbl)
            n163 = Divide(x=w422, y=w381) -> (x/y=w423:dbl)
            n164 = Divide(x=w423, y=w375) -> (x/y=w424:dbl)
            n165 = call <instrlib>:"niFgen Set Sample Rate.vi"("error in (no error)"=w404, "Sample Rate (Samp/s)"=w423, "Instrument Handle"=w403) -> ("error out"=w323:errorcluster, "Instrument Handle Out"=w320:refnum<k15>)  [unwired: 7 in]
            n166 = call <instrlib>:"niFgen Set Sample Rate.vi"("error in (no error)"=w406, "Sample Rate (Samp/s)"=w424, "Instrument Handle"=w405) -> ("error out"=w435:errorcluster, "Instrument Handle Out"=w393:refnum<k15>)  [unwired: 7 in]
            n167 = call <instrlib>:"niFgen Allocate Waveform.vi"("error in (no error)"=w323, "Waveform Size"=w319, "Instrument Handle"=w320) -> ("error out"=w322:errorcluster, "Waveform Handle Out"=w317:i32, "Instrument Handle Out"=w321:refnum<k15>)  [unwired: 6 in]
            n168 = property class="niFgen"(reference=w321, error in=w322, "Load Impedance"=w421, "Gain"=w383) -> (reference out=w327:refnum<k15>, error out=w324:errorcluster, "Sample Rate"=w345:dbl)
            n169 = local read "X single line pattern"() -> (w318:dbl[])
            n170 = Multiply(x=w355, y=w376) -> (x*y=w354:u32)
            n171 = Reshape Array(w426, w354) -> (w427:dbl[])
            n172 = case shown="False" w353 {
              tunnel: w393 -> [w454 w462]
              tunnel: w421 -> [w453 w463]
              tunnel: w427 -> [w452 _]
              tunnel: [w451 _] -> w358
              tunnel: [w450 w458] -> w438
              tunnel: [w449 w457] -> w439
              tunnel: w435 -> [w444 w461]
              tunnel: w349 -> [w442 _]
              tunnel: w383 -> [w440 w456]
              frame False {
                w443 = 1 items=["NIFGEN_VAL_SINGLE"=1, "NIFGEN_VAL_CONTINUOUS"=2, "NIFGEN_VAL_STEPPED"=3, "NIFGEN_VAL_BURST"=4] ("Triggers:Trigger Mode")
                n173 = call <instrlib>:"niFgen Allocate Waveform.vi"("error in (no error)"=w444, "Waveform Size"=w442, "Instrument Handle"=w454) -> ("error out"=w445:errorcluster, "Waveform Handle Out"=w451:i32, "Instrument Handle Out"=w448:refnum<k15>)  [unwired: 6 in]
                n174 = local read "Repeat count"() -> (w441:u32)
                n175 = property class="niFgen"(reference=w448, error in=w445, "Load Impedance"=w453, "Gain"=w440, "Streaming Waveform Handle"=w451, "Repeat Count"=w441, "Trigger Mode"=w443) -> (reference out=w447:refnum<k15>, error out=w446:errorcluster)
                n176 = call-poly <instrlib>:"niFgen Write Waveform (poly).vi"("Waveform Data"=w452, "error in (no error)"=w446, "Waveform Handle"=w451, "Instrument Handle"=w447) -> ("error out"=w449:errorcluster, "Instrument Handle Out"=w450:refnum<k15>)  [unwired: 5 in, 1 out]
              }
              frame True {
                n177 = property class="niFgen"(reference=w462, error in=w461, "Load Impedance"=w463, "Gain"=w456) -> (reference out=w460:refnum<k15>, error out=w459:errorcluster)
                n178 = local read "Y scan pattern"() -> (w455:dbl[])
                n179 = call-poly <instrlib>:"niFgen Create Waveform (poly).vi"("error in (no error)"=w459, "Waveform Data Array"=w455, "Instrument Handle"=w460) -> ("error out"=w457:errorcluster, "Instrument Handle Out"=w458:refnum<k15>)  [unwired: 6 in, 1 out]
              }
            }
            n180 = call-poly <instrlib>:"niFgen Write Waveform (poly).vi"("Waveform Data"=w318, "error in (no error)"=w324, "Waveform Handle"=w317, "Instrument Handle"=w327) -> ("error out"=w325:errorcluster, "Instrument Handle Out"=w326:refnum<k15>)  [unwired: 5 in, 1 out]
            n181 = call <instrlib>:"niScope Get Session Reference.vi"("instrument handle"=w413, "error in"=w415) -> ("instrument handle out"=w362:refnum<k15>, "session reference"=w428:refnum<k20>, "error out"=w366:errorcluster)  [unwired: 11 in]
            n182 = call <instrlib>:"niFgen Get Session Reference.vi"("error in (no error)"=w325, "Instrument Handle"=w326) -> ("error out"=w369:errorcluster, "Session Reference"=w430:refnum<k20>, "Instrument Handle Out"=w365:refnum<k15>)  [unwired: 7 in]
            n183 = call <instrlib>:"niFgen Get Session Reference.vi"("error in (no error)"=w439, "Instrument Handle"=w438) -> ("error out"=w367:errorcluster, "Session Reference"=w429:refnum<k20>, "Instrument Handle Out"=w363:refnum<k15>)  [unwired: 7 in]
            n184 = Build Array(w430, w429, w428) -> (w372:refnum<k20>[])
            n185 = call <instrlib>:"niTClk Configure For Homogeneous Triggers.vi"("error in (no error)"=w369, "sessions"=w372) -> ("error out"=w370:errorcluster, "sessions out"=w371:refnum<k20>[])  [unwired: 8 in]
            n186 = call <instrlib>:"niTClk Synchronize.vi"("error in (no error)"=w370, "sessions"=w371) -> ("error out"=w368:errorcluster, "sessions out"=w364:refnum<k20>[])  [unwired: 8 in]
            n187 = Merge Errors(w368, w367, w366) -> (w361:errorcluster)
            n188 = local read "AO SampClk.MaxRate"() -> (w357:dbl)
            n189 = local read "AI SampClk.MaxRate"() -> (w356:dbl)
            n190 = local read "Scan speed"() -> (w340:u8)
            n191 = local read "Detector number"() -> (w330:u8)
            n192 = local read "X min (V)"() -> (w334:dbl)
            n193 = local read "X max (V)"() -> (w333:dbl)
            n194 = local read "X min index"() -> (w332:i32)
            n195 = local read "X max index"() -> (w331:i32)
            n196 = local read "Y min (V)"() -> (w329:dbl)
            n197 = local read "Y max (V)"() -> (w328:dbl)
            n198 = local read "AO multiline"() -> (w339:u32)
            n199 = local read "Decimating factor"() -> (w338:u16)
            n200 = local read "Total time"() -> (w337:dbl)
            n201 = local read "Scan time (m)"() -> (w336:dbl)
            n202 = local read "Scan time (s)"() -> (w335:dbl)
            n203 = local read "X resolution"() -> (w344:u32)
            n204 = local read "Y resolution"() -> (w343:u32)
            n205 = local read "X resolution with rampdown"() -> (w342:i32)
            n206 = local read "Oversampling"() -> (w341:u32)
            n207 = local read "Waveform blocks"() -> (w347:u32)
            n208 = local read "Repeat count"() -> (w348:u32)
            n209 = local read "Initialized handles"() -> (w360:T2)
            n210 = Bundle By Name(cluster=w360, "sessions out"=w364, "SEM-X handle out"=w365, "SEM-Y handle out"=w363, "SEM-Y waveform handle out"=w358, "Detectors handle out"=w362, "channels"=w346, "error out"=w361, "Others.AO SampClk.MaxRate"=w357, "Others.AI SampClk.MaxRate"=w356, "Others.AO rate"=w345, "Others.Scan speed"=w340, "Others.Detector number"=w330, "Others.X min (V)"=w334, "Others.X max (V)"=w333, "Others.X min index"=w332, "Others.X max index"=w331, "Others.Y min (V)"=w329, "Others.Y max (V)"=w328, "Others.AO multiline"=w339, "Others.Decimating factor"=w338, "Others.Total time"=w337, "Others.Scan time (m)"=w336, "Others.Scan time (s)"=w335, "Others.X resolution"=w344, "Others.Y resolution"=w343, "Others.X resolution with rampdown"=w342, "Others.Oversampling"=w341, "Others.Y scan pts per line"=w355, "Others.Y scan pts per AO multiline"=w354, "Others.Small scan"=w353, "Others.Y single line pattern"=w352, "Others.Detectors min record length"=w351, "Others.Waveform blocks"=w347, "Others.Repeat count"=w348, "Others.Waveform size"=w349, "Others.AI multiline"=w350) -> (w359:T2)
          }
        }
      }
      frame "Get Reference" {
        w557 = 64 ("y")
        w519 = 10.0 ("x")
        n211 = Unbundle By Name(w524) -> ("Detectors handle out"=w522:refnum<k15>)
        n212 = Unbundle By Name(w524) -> ("SEM-X handle out"=w481:refnum<k15>, "Others.AO rate"=w496:dbl, "Others.X resolution with rampdown"=w497:i32, "error out"=w503:errorcluster)
        n213 = Unbundle By Name(w527) -> ("X resolution"=w553:u32, "Y resolution"=w542:u32, "X center (um)"=w547:dbl, "Y center (um)"=w549:dbl, "X size (V)"=w551:dbl, "Scan rate (Hz)"=w486:u32, "Frame line rampdown ratio"=w540:sgl, "Pixel size (nm)"=w552:sgl)  [unwired: 2 out]
        n214 = Unbundle By Name(w524) -> ("Others.Y max (V)"=w510:dbl, "Others.Y scan pts per line"=w516:i32, "Others.AO multiline"=w517:u32, "Others.Y scan pts per AO multiline"=w514:i32, "SEM-Y handle out"=w560:refnum<k15>, "SEM-Y waveform handle out"=w563:i32, "error out"=w559:errorcluster, "Others.Small scan"=w512:bool)
        n215 = Not Equal?(x=w522, y=refnum<k15> refnum ("Detectors handle out")) -> (x != y?=w520:bool)
        n216 = Multiply(x=w553, y=w552) -> (x*y=w544:sgl)
        n217 = case shown="True" w520 {
          tunnel: w522 -> [_ w578]
          tunnel: [FALSE w577] -> w521
          frame False {
          }
          frame True {
            n218 = property class="niScope"(reference=w578) -> (error out=w576:errorcluster, "Actual Sample Rate"=w579:dbl)  [unwired: 1 in, 1 out]
            n219 = Not Equal To 0?(x=w579) -> (x != 0?=w577:bool)
            n220 = call <vilib>:"Clear Errors.vi"("error in (no error)"=w576) -> ()  [unwired: 5 in, 2 out]
          }
        }
        n221 = expression code="x/1000"(w544) -> (w545:sgl)
        n222 = Divide(x=w545, y=w551) -> (x/y=w548:dbl)
        n223 = local read "AO SampClk.MaxRate"() -> (w480:dbl)
        n224 = Divide(x=w547, y=w548) -> (x/y=w546:dbl)
        n225 = Divide(x=w549, y=w548) -> (x/y=w550:dbl)
        n226 = Multiply(x=w551, y=w542) -> (x*y=w541:dbl)
        n227 = Divide(x=w541, y=w553) -> (x/y=w543:dbl)
        n228 = expression code="x/2"(w551) -> (w531:dbl)
        n229 = expression code="x/2"(w543) -> (w530:dbl)
        n230 = In Range and Coerce(upper limit=w480, x=w486, lower limit=u32 10000) -> (coerced(x)=w488:dbl)  [unwired: 1 out]
        n231 = Add(x=w546, y=w531) -> (x+y=w533:dbl)
        n232 = Subtract(x=w546, y=w531) -> (x-y=w532:dbl)
        n233 = Subtract(x=w550, y=w530) -> (x-y=w534:dbl)
        n234 = Add(x=w550, y=w530) -> (x+y=w535:dbl)
        n235 = call <instrlib>:"niFgen Clear Arbitrary Memory.vi"("error in (no error)"=w503, "Instrument Handle"=w481) -> ("error out"=w505:errorcluster, "Instrument Handle Out"=w504:refnum<k15>)  [unwired: 8 in]
        n236 = Divide(x=w488, y=1000000.0) -> (x/y=w493:dbl)
        n237 = Divide(x=w533, y=w519) -> (x/y=w537:dbl)
        n238 = Divide(x=w532, y=w519) -> (x/y=w536:dbl)
        n239 = Divide(x=w534, y=w519) -> (x/y=w538:dbl)
        n240 = Divide(x=w535, y=w519) -> (x/y=w539:dbl)
        n241 = call <instrlib>:"niFgen Set Sample Rate.vi"("error in (no error)"=w505, "Sample Rate (Samp/s)"=w496, "Instrument Handle"=w504) -> ("error out"=w501:errorcluster, "Instrument Handle Out"=w502:refnum<k15>)  [unwired: 7 in]
        n242 = expression code="log2(x)"(w493) -> (w491:dbl)
        n243 = Round Toward -Infinity(1:w491) -> (0:w492:dbl)
        n244 = Scale By Power Of 2(n=w492, x=ext 1.0) -> (x*2^n=w494:ext)
        n245 = call <instrlib>:"niFgen Allocate Waveform.vi"("error in (no error)"=w501, "Waveform Size"=w497, "Instrument Handle"=w502) -> ("error out"=w499:errorcluster, "Waveform Handle Out"=w498:i32, "Instrument Handle Out"=w500:refnum<k15>)  [unwired: 6 in]
        n246 = Round Toward +Infinity(x=w494) -> (ceil(x): smallest int >= x=w495:ext)
        n247 = To Unsigned Byte Integer(number=w495) -> (unsigned 8bit integer=w483:u8)
        n248 = In Range and Coerce(upper limit=u8 255 ("X round to"), x=w483, lower limit=u8 4 ("X round to")) -> (coerced(x)=w482:u8)  [unwired: 1 out]
        n249 = call "Raster scan.vi"("X resolution"=w553, "X round to"=w482, "Frame line rampdown ratio"=w540, "Y resolution"=w542, "X start"=w536, "Y start"=w538, "X end"=w537, "Y end"=w539) -> ("X single line pattern"=w506:dbl[], "Y single line pattern"=w528:dbl[])  [unwired: 4 in, 6 out]
        n250 = Array Size(array=w528) -> (size(s)=w554:i32)
        n251 = Quotient & Remainder(x=w554, y=w557) -> (x-y*floor(x/y)=w558:i32)  [unwired: 1 out]
        n252 = Subtract(x=w557, y=w558) -> (x-y=w556:i32)
        n253 = Multiply(x=w519, y=w528) -> (x*y=w529:dbl[])
        n254 = for {
          N: w556 -> [_]
          tunnel: [1.0 ("x")] -> w555 mode=indexing
        }
        n255 = Array Max & Min(array=w529) -> (max value=w511:dbl, min value=w526:dbl)  [unwired: 2 out]
        n256 = call-poly <instrlib>:"niFgen Write Waveform (poly).vi"("Waveform Data"=w506, "error in (no error)"=w499, "Waveform Handle"=w498, "Instrument Handle"=w500) -> ("error out"=w507:errorcluster, "Instrument Handle Out"=w508:refnum<k15>)  [unwired: 5 in, 1 out]
        n257 = Build Array (concatenate)(w528, w555) -> (w513:dbl[])
        n258 = case shown="False" w512 {
          tunnel: w511 -> [_ w571]
          tunnel: w510 -> [_ w570]
          tunnel: [TRUE w569] -> w509
          frame False {
          }
          frame True {
            n259 = Equal?(x=w571, y=w570) -> (x = y?=w569:bool)
          }
        }
        n260 = for {
          N: w517 -> [_]
          tunnel: [w574] -> w518 mode=indexing
          tunnel: w513 -> [w573] mode=indexing
          tunnel: w516 -> [w572]
          n261 = Initialize Array(w573, w572) -> (w574:dbl[])
        }
        n262 = Compound Arithmetic op=AND(w521, w520, w509) -> (→"Tclk handle valid":bool)
        n263 = local read "X resolution"() -> (w477:u32)
        n264 = local read "Image fit to"() -> (w479:u8)
        n265 = local read "Y resolution"() -> (w478:u32)
        n266 = Reshape Array(w518, w514) -> (w515:dbl[])
        n267 = case shown="False" w512 {
          tunnel: w560 -> [w583 w588]
          tunnel: [w586 w588] -> w564
          tunnel: [w585 w587] -> w562
          tunnel: w559 -> [w582 w587]
          tunnel: w563 -> [w584 _]
          tunnel: w515 -> [w581 _]
          frame False {
            n268 = call-poly <instrlib>:"niFgen Write Waveform (poly).vi"("Waveform Data"=w581, "error in (no error)"=w582, "Waveform Handle"=w584, "Instrument Handle"=w583) -> ("error out"=w585:errorcluster, "Instrument Handle Out"=w586:refnum<k15>)  [unwired: 5 in, 1 out]
          }
          frame True {
          }
        }
        n269 = case shown="0, Default" w479 {
          tunnel: w477 -> [w566 _]
          tunnel: w478 -> [_ w567]
          tunnel: [w566 w567] -> w473
          frame 0, Default {
          }
          frame 1 {
          }
        }
        n270 = Merge Errors(w507, w562) -> (w561:errorcluster)
        n271 = Quotient & Remainder(x=w473, y=u32 512) -> (floor(x/y)=w475:u32)  [unwired: 1 out]
        n272 = To Unsigned Word Integer(number=w475) -> (unsigned 16bit integer=w471:u16)
        n273 = In Range and Coerce(upper limit=u16 100, x=w471, lower limit=u16 1) -> (coerced(x)=w470:u16)  [unwired: 1 out]
        n274 = Bundle By Name(cluster=w524, "Others.Decimating factor"=w470, "SEM-X handle out"=w508, "SEM-Y handle out"=w564, "error out"=w561, "Others.Y min (V)"=w526, "Others.Y max (V)"=w511, "Others.Y single line pattern"=w513) -> (w565:T2)
      }
      frame "Close Reference" {
        n275 = Unbundle By Name(w597) -> ("SEM-X handle out"=w596:refnum<k15>, "SEM-Y handle out"=w595:refnum<k15>, "Detectors handle out"=w593:refnum<k15>, "error out"=w592:errorcluster)
        n276 = Build Array(w596, w595) -> (w594:refnum<k15>[])
        n277 = call <instrlib>:"niScope Abort.vi"("instrument handle"=w593, "error in"=w592) -> ("instrument handle out"=w590:refnum<k15>, "error out"=w591:errorcluster)  [unwired: 12 in]
        n278 = call <instrlib>:"niScope Close.vi"("instrument handle"=w590, "error in"=w591) -> ("error out"=w589:errorcluster)  [unwired: 13 in]
        n279 = for {
          tunnel: w594 -> [w607] mode=indexing
          shift-right: [w604] -> _
          shift-left: w589 -> [w606]
          n280 = call <instrlib>:"niFgen Abort Generation.vi"("error in (no error)"=w606, "Instrument Handle"=w607) -> ("error out"=w605:errorcluster, "Instrument Handle Out"=w603:refnum<k15>)  [unwired: 8 in]
          n281 = call <instrlib>:"niFgen Close.vi"("error in (no error)"=w605, "Instrument Handle"=w603) -> ("error out"=w604:errorcluster)  [unwired: 9 in]
        }
        n282 = Bundle By Name(cluster=w597, "sessions out"=refnum<k20>[] [], "SEM-X handle out"=refnum<k15> refnum ("Instrument Handle Out"), "SEM-Y handle out"=refnum<k15> refnum ("Instrument Handle Out"), "Detectors handle out"=refnum<k15> refnum ("instrument handle out")) -> (w598:T2)
      }
    }
  }
  "Initialized handles" <- w7
  n283 = shared-variable ".\\Zeiss Library.lvlib\\Tclk para"(w5) -> ()  [unwired: 1 in, 1 out]
